vi "Main.vi"() -> ()   [LabVIEW 2017]
uses:
  type defs/action buttons.ctl
  type defs/mode buttons.ctl
  <vilib>/vision/Pattern Matching.llb/IMAQ GM Match Report.ctl
  type defs/states.ctl
  type defs/data.ctl
  <vilib>/vision/Image Controls.llb/IMAQ Image.ctl
  <vilib>/myRIO/Instrument Drivers/Onboard IO/PWM/typedefs/PWM Reference.ctl
  <vilib>/myRIO/Common/Instrument Driver Framework/Utilities/typedefs/myRIO Generic Hardware Reference.ctl
  <vilib>/myRIO/Common/Instrument Driver Framework/Utilities/typedefs/Hardware Version Enum.ctl
  <vilib>/myRIO/Common/Instrument Driver Framework/Utilities/typedefs/myRIO v1.0 Reference.ctl
  <vilib>/myRIO/Common/Instrument Driver Framework/Utilities/typedefs/Generic FPGA Reference.ctl
  <vilib>/myRIO/Common/Instrument Driver Framework/myRIO v1.0/PWM/typedefs/PWM Channels Enum.ctl
  <vilib>/myRIO/Instrument Drivers/Onboard IO/PWM/typedefs/PWM Configuration.ctl
  <vilib>/userdefined/High Color/nirio_resource_hc.ctl
  <vilib>/myRIO/Instrument Drivers/Onboard IO/DIO/typedefs/DIO Reference.ctl
  <vilib>/myRIO/Common/Instrument Driver Framework/myRIO v1.0/DIO/typedefs/DIO Channels List.ctl
  <vilib>/myRIO/Common/Instrument Driver Framework/myRIO v1.0/DIO/typedefs/DIO Channels Enum.ctl
  type defs/task.ctl
  <vilib>/myRIO/Common/Instrument Driver Framework/Utilities/vis/Is FPGA Ref Available.vi
  <vilib>/myRIO/Common/Instrument Driver Framework/myRIO v1.0/PWM/vis/myRIO v1.1 Open PWM.vi
  <vilib>/myRIO/Instrument Drivers/Onboard IO/PWM/vis/Set Duty Cycle and Frequency.vi
  <vilib>/myRIO/Common/Instrument Driver Framework/myRIO v1.0/DIO/vis/myRIO v1.1 Open DIO.vi
  <vilib>/myRIO/Instrument Drivers/Onboard IO/DIO/vis/Write.vi
  <vilib>/myRIO/Instrument Drivers/Onboard IO/DIO/vis/Read.vi
  <vilib>/myRIO/Common/Instrument Driver Framework/Utilities/vis/Validate Channels.vi
  <vilib>/myRIO/Common/Instrument Driver Framework/myRIO v1.0/PWM/vis/myRIO v1.0 Reserve PWM.vi
  <vilib>/myRIO/Common/Instrument Driver Framework/myRIO v1.0/DIO/vis/myRIO v1.0 Reserve DIO.vi
  <vilib>/myRIO/Common/Instrument Driver Framework/myRIO v1.0/UART/vis/myRIO v1.0 Close UART.vi
  <vilib>/myRIO/Common/Instrument Driver Framework/myRIO v1.0/PWM/vis/myRIO v1.0 Build MUX Configuration PWM.vi
  <vilib>/myRIO/Common/Instrument Driver Framework/myRIO v1.0/Resource Manager/vis/myRIO v1.0 Reserve Channel List.vi
  <vilib>/myRIO/Common/Instrument Driver Framework/myRIO v1.0/DIO/vis/myRIO v1.0 Build MUX Configuration DIO.vi
  <vilib>/myRIO/Common/Instrument Driver Framework/myRIO v1.0/Resource Manager/vis/myRIO v1.0 Create Configuration List.vi
  <vilib>/myRIO/Common/Instrument Driver Framework/myRIO v1.0/Resource Manager/vis/myRIO v1.0 Reserve Channel.vi
  <vilib>/myRIO/Common/Instrument Driver Framework/myRIO v1.0/Resource Manager/vis/myRIO v1.0 Unreserve Channel.vi
  <vilib>/myRIO/Common/Instrument Driver Framework/myRIO v1.0/Resource Manager/vis/myRIO v1.0 Build Mutex Name.vi
  <vilib>/Utility/VariantDataType/GetNumericInfo.vi
  <vilib>/Utility/error.llb/Error Cluster From Error Code.vi
  <vilib>/myRIO/Common/Instrument Driver Framework/myRIO v1.0/myRIO v1.1 Open.vi
  <vilib>/myRIO/Common/Instrument Driver Framework/Utilities/vis/IO Manager.vi
  <vilib>/myRIO/Common/Instrument Driver Framework/Utilities/vis/Configuration Manager.vi
  <vilib>/myRIO/Common/Instrument Driver Framework/myRIO v1.0/Resource Manager/vis/myRIO v1.0 Configure IO.vi
  <vilib>/myRIO/Common/Instrument Driver Framework/myRIO v1.0/myRIO v1.0 Close.vi
  <vilib>/myRIO/Common/Instrument Driver Framework/myRIO v1.0/PWM/vis/myRIO v1.0 Write PWM.vi
  <vilib>/myRIO/Common/Instrument Driver Framework/myRIO v1.0/DIO/vis/myRIO v1.0 Write DIO.vi
  <vilib>/myRIO/Common/Instrument Driver Framework/myRIO v1.0/DIO/vis/myRIO v1.0 Read DIO.vi
  <vilib>/myRIO/Common/Instrument Driver Framework/Utilities/vis/FPGA Ref Manager.vi
  <vilib>/myRIO/Common/Instrument Driver Framework/myRIO v1.0/myRIO v1.0 Reset FPGA.vi
  <vilib>/myRIO/Common/Instrument Driver Framework/myRIO v1.0/IRQ/vis/myRIO v1.0 IRQ Info FGV.vi
  <vilib>/myRIO/Common/Instrument Driver Framework/myRIO v1.0/IRQ/vis/myRIO v1.0 Timer IRQ Info FGV.vi
  <vilib>/myRIO/Common/Instrument Driver Framework/myRIO v1.0/IRQ/vis/myRIO v1.0 ISR Agent.vi
  <vilib>/myRIO/Express VI/Onboard IO/PWM/PWM Express VI.xnode
  <vilib>/myRIO/Instrument Drivers/Onboard IO/PWM/vis/myRIO PWM Open.xnode
  <vilib>/myRIO/Express VI/Onboard IO/DO/DO Express VI.xnode
  <vilib>/myRIO/Instrument Drivers/Onboard IO/DIO/vis/myRIO DIO Open.xnode
  <vilib>/myRIO/Express VI/Onboard Devices/LED/LED Express VI.xnode
  <vilib>/myRIO/Express VI/Onboard Devices/Button/Button Express VI.xnode
  <vilib>/vision/NI_Vision_Development_Module.lvlib
  <vilib>/myRIO/Instrument Drivers/Onboard IO/DIO/DIO.lvlib
  <vilib>/myRIO/Instrument Drivers/Onboard IO/PWM/PWM.lvlib
  <vilib>/myRIO/Instrument Drivers/Utilities/Utilities.lvlib
panel:
  in  "ROI Descriptor COLOR":T1={"Global Rectangle"=[86, 71, 180, 164], "Contours"=[{"ID"=enum."External", "Type"=3, "Coordinates"=[86, 71, 180, 164]}]} {"Contours"."Type" items=["No Selection", "Point", "Line", "Rectangle", "Oval", "Polygon", "Freehand Region", "Annulus", "Unused2", "Unused3", "Broken Line", "Freehand Line", "Rotated Rectangle"]}
  out "y0 (circle)":i32
  out "x0 (circle)":i32
  out "x1 (circle)":i32
  out "y1 (circle)":i32
  in  "divider (circle)":dbl=1.0
  out "error out 2":errorcluster
  out "___Test___":i32[](array[numeric])
  in  "Ball index":i32=1
  out "CircleRadius":dbl
  in  "Look at ball":bool
  in  "x = y?":bool
  in  "y":sgl=1.0
  out "Scale":sgl
  out "error out":errorcluster
  in  "Tab Control":enum32{"Motors", "Shape/Color", "Pattern"}(tab)
  in  "Left+":bool
  in  "Left-":bool
  in  "Right+":bool
  in  "Right-":bool
  in  "M+":bool
  in  "M-":bool
  in  "G+":bool
  in  "G-":bool
  in  "M_PWM":dbl=0.5
  in  "L_PWM":dbl=0.5
  in  "R_PWM":dbl=0.5
  in  "M+ (onGrab)":bool
  out "Circles Calibrated (Shape Detection 1)":T2(array[cluster]) {"Position"."Y" format="%.2f"; "Position"."X" format="%.2f"}
  out "Number of Matches (Shape Detection 1)":i32
  out "Color":i32
  in  "Circle Descriptor (Shape Detection 1)":cluster{"Min Radius":dbl, "Max Radius":dbl}={"Min Radius"=16.0, "Max Radius"=500.0}
  in  "Align X - t, Y - f":bool
  in  "grab time (ms)":u32
  out "Class (Particle Classification 1)":string
  out "y0":i32
  out "x0":i32
  out "x1":i32
  out "y1":i32
  out "Number of Matches (Geometric Matching 1)":i32
  out "Calibrated Matches (Geometric Matching 1)":T3[](array[typedef]) {"Correlation Score" format="%.2f"; "Target Template Curve Score" format="%.2f"; "Template Target Curve Score" format="%.2f"; "Bounding Box"."y" format="%.2f"; "Bounding Box"."x" format="%.2f"; "Position"."y" format="%.2f"; "Position"."x" format="%.2f"; "Score" format="%.2f"; "Scale" format="%.2f"; "Angle" format="%.2f"; "Occlusion %" format="%.2f"}
  out "curY":dbl
  out "curX":dbl
  out "Y is in range":bool
  out "X is in range":bool
  in  "defY":dbl=170.0
  in  "Range":dbl=40.0
  in  "defX":dbl=150.0
  in  "mode buttons":T4
  out "image display":T5(plugin-control)
  in  "action buttons":T6
  in  "Stop":bool
  # "Machine\nVision\nApp"
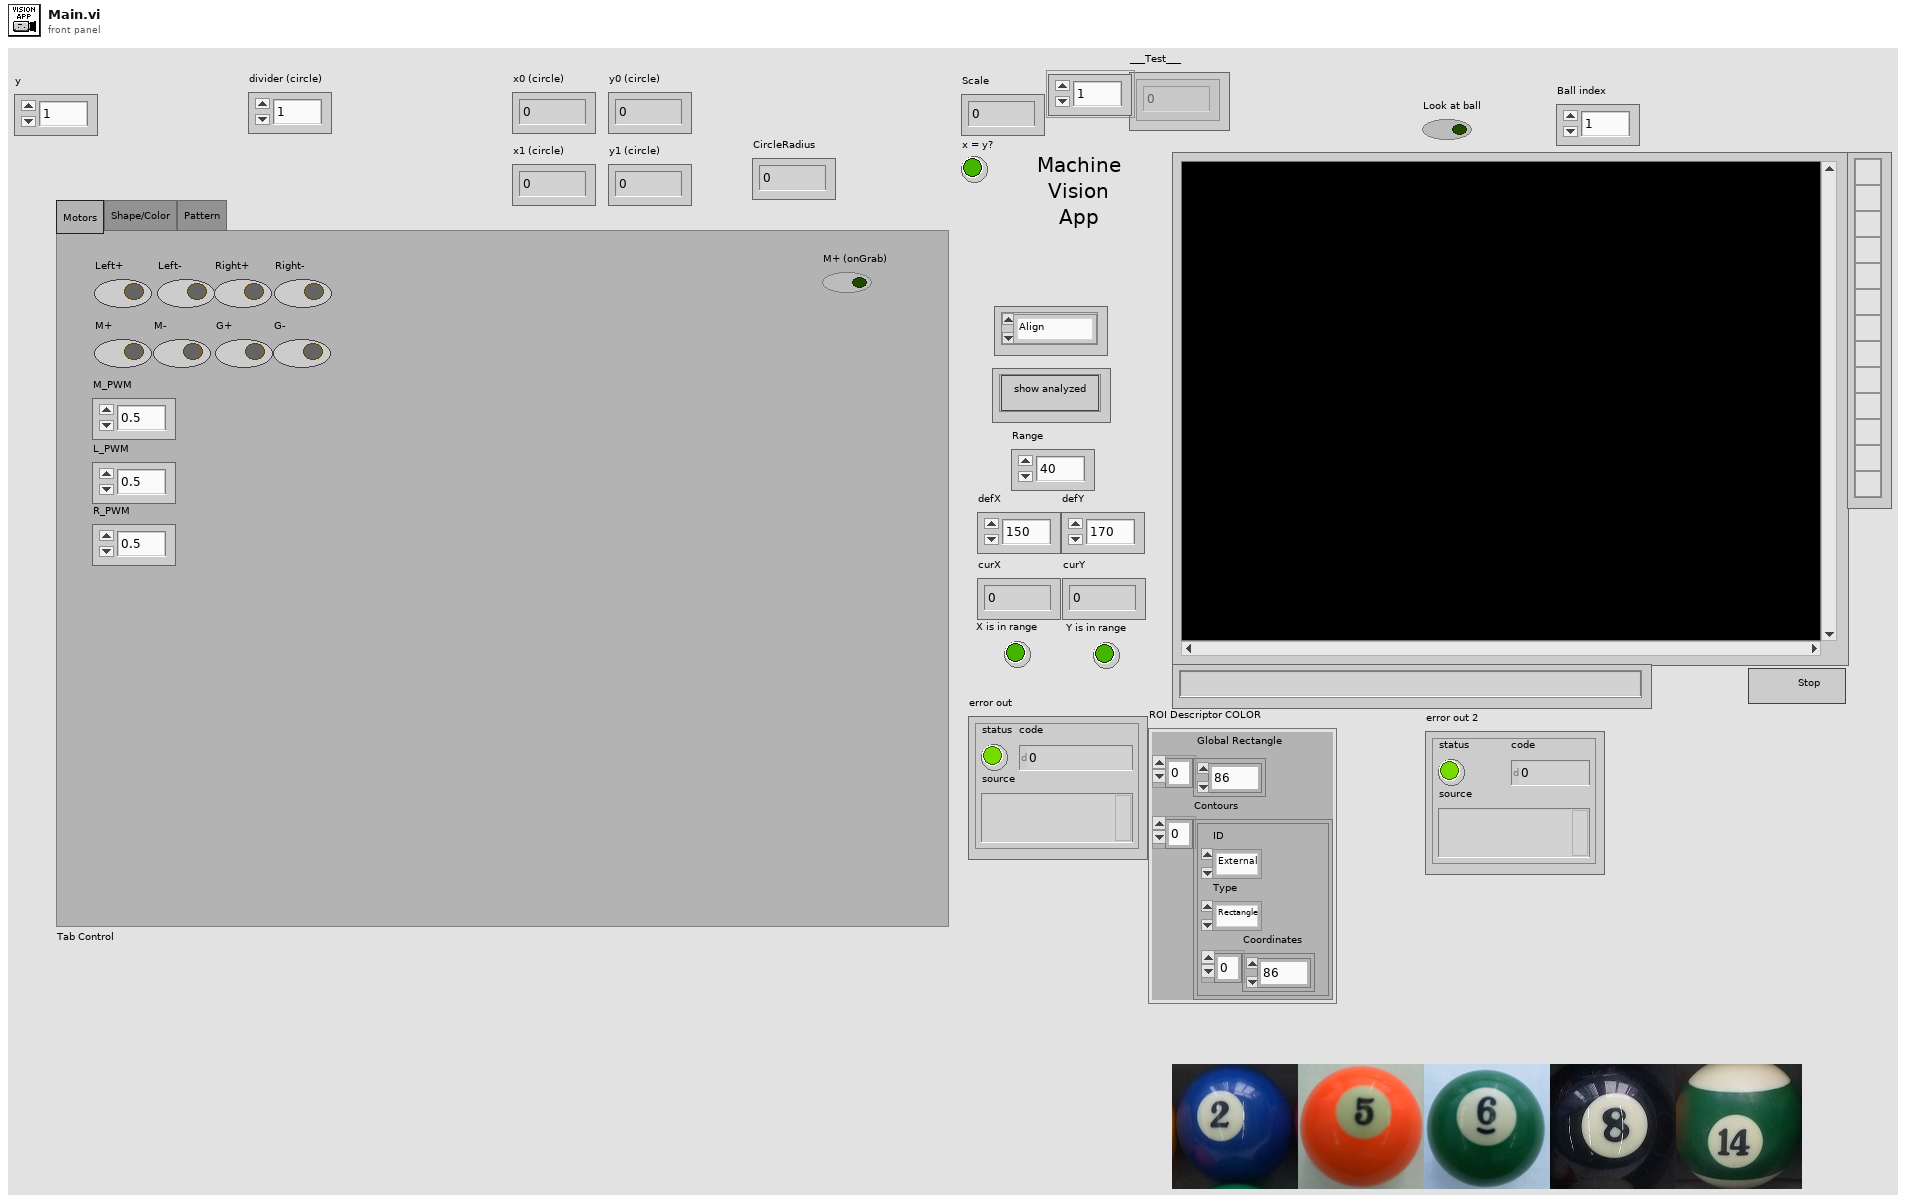
[diagram p1: front panel]
types:
  T1 = cluster{"Global Rectangle":i32[], "Contours":cluster{"ID":enum32{"External", "Internal"}, "Type":u32, "Coordinates":i32[]}[]}
  T2 = cluster{"Position":cluster{"X":sgl, "Y":sgl}, "Radius":dbl, "Score":dbl}[]
  T3 = typedef "IMAQ GM Match Report.ctl" = cluster{"Position":cluster{"x":sgl, "y":sgl}, "Angle":sgl, "Scale":sgl, "Score":sgl, "Bounding Box":cluster{"x":sgl, "y":sgl}[], "Contrast Reversed":bool, "Occlusion %":sgl, "Template Target Curve Score":sgl, "Target Template Curve Score":sgl, "Correlation Score":sgl}
  T4 = typedef "mode buttons.ctl" = cluster{"show analyzed":bool}
  T5 = typedef "IMAQ Image.ctl" = refnum<image>
  T6 = typedef "action buttons.ctl" = cluster{"Shape - t, Color - f":enum16{"Align", "Pattern", "Ball", "Other", "Clear", "Joystick control"}}
  T7 = typedef "data.ctl" = cluster{"Shape - t, Color - f":bool, "qsm":cluster{"Webcam image ref":T5, "Analyzed image ref":T5, "Stop webcam":bool}, " image ref":T5, "number img":i32, "ROI Descriptor (Image Mask 1)":cluster{"Global Rectangle":i32[], "Contours":cluster{"ID":enum32{"External", "Internal"}, "Type":u32, "Coordinates":i32[]}[]}, "Pattern class":i32, "Color class":i32, "ROI Descriptor COLOR Mask":cluster{"Global Rectangle":i32[], "Contours":cluster{"ID":enum32{"External", "Internal"}, "Type":u32, "Coordinates":i32[]}[]}, "___Test___":i32[], "ball Positions":i32[]}
  T8 = typedef "states.ctl" = enum16{"(qsm) schedule", "(qsm) initialize", "(qsm) release", "(qsm) clean up", "(qsm) shutdown", "(myRIO) initialize", "(myRIO) clean up", "(myRIO) update ports", "(image) get", "(image) analyze", "(image) show", "(ball) Shape detection", "(ball) Calc ball indx", "(ball) Calculate ROI", "X align", "Wait", "Grab", "(pattern) Find Square", "(pattern) Calculate ROI", "(pattern) Analyze pattern", "(joystick) Joystick control", "Wait for button"}
  T9 = typedef "DIO.lvlib/DIO Reference.ctl" = cluster{"myRIO Reference":T10, "DIO Channels List":T14}
  T10 = typedef "myRIO Generic Hardware Reference.ctl" = cluster{"myRIO Model":T11, "myRIO Hardware Reference":T12}
  T11 = typedef "Hardware Version Enum.ctl" = enum16{"Unknown", "myRIO-1900", "myRIO-1950", "roboRIO", "NI ELVIS RIO CM"}
  T12 = typedef "myRIO v1.0 Reference.ctl" = cluster{"Generic FPGA Reference":T13, "Allow multiple opens":bool}
  T13 = typedef "Generic FPGA Reference.ctl" = refnum<k20>
  T14 = typedef "DIO Channels List.ctl" = T15[]
  T15 = typedef "DIO Channels Enum.ctl" = enum16{"Not Connected", "C/DIO0", "C/DIO1", "C/DIO2", "C/DIO3", "C/DIO4", "C/DIO5", "C/DIO6", "C/DIO7", "A/DIO0", "A/DIO1", "A/DIO2", "A/DIO3", "A/DIO4", "A/DIO5", "A/DIO6", "A/DIO7", "A/DIO8", "A/DIO9", "A/DIO10", "A/DIO11", "A/DIO12", "A/DIO13", "A/DIO14", "A/DIO15", "B/DIO0", "B/DIO1", "B/DIO2", "B/DIO3", "B/DIO4", "B/DIO5", "B/DIO6", "B/DIO7", "B/DIO8", "B/DIO9", "B/DIO10", "B/DIO11", "B/DIO12", "B/DIO13", "B/DIO14", "B/DIO15", "LED0", "LED1", "LED2", "LED3", "Button0", "DIO/DIO0", "DIO/DIO1", "DIO/DIO2", "DIO/DIO3", "DIO/DIO4", "DIO/DIO5", "DIO/DIO6", "DIO/DIO7", "DIO/DIO8", "DIO/DIO9", "SPI/CS0", "SPI/CS1", "SPI/CS2", "SPI/CS3", "LED RADIO (Green)", "LED RADIO (Red)", "LED COMM (Green)", "LED COMM (Red)", "LED MODE (Green)", "LED MODE (Red)"}
  T16 = typedef "nirio_resource_hc.ctl" = tag
  T17 = typedef "PWM.lvlib/PWM Reference.ctl" = cluster{"myRIO Reference":T10, "PWM Channels Enum":T18, "PWM Configuration":T19}
  T18 = typedef "PWM Channels Enum.ctl" = enum16{"Not Connected", "C/PWM0", "C/PWM1", "A/PWM0", "A/PWM1", "A/PWM2", "B/PWM0", "B/PWM1", "B/PWM2", "PWM/PWM0", "PWM/PWM1", "PWM/PWM2", "PWM/PWM3", "PWM/PWM4", "PWM/PWM5", "PWM/PWM6", "PWM/PWM7", "PWM/PWM8", "PWM/PWM9"}
  T19 = typedef "PWM.lvlib/PWM Configuration.ctl" = cluster{"Frequency":dbl, "Duty Cycle":dbl}
  T20 = enum16{"Align", "Pattern", "Ball", "Other", "Clear", "Joystick control"}
  T21 = typedef "task.ctl" = T8[]
  T22 = typedef "Image Type" = u32
  T23 = cluster{"Position":cluster{"X":sgl, "Y":sgl}, "Radius":dbl, "Score":dbl}
  T24 = cluster{"ID":enum32{"External", "Internal"}, "Type":u32, "Coordinates":i32[]}[]
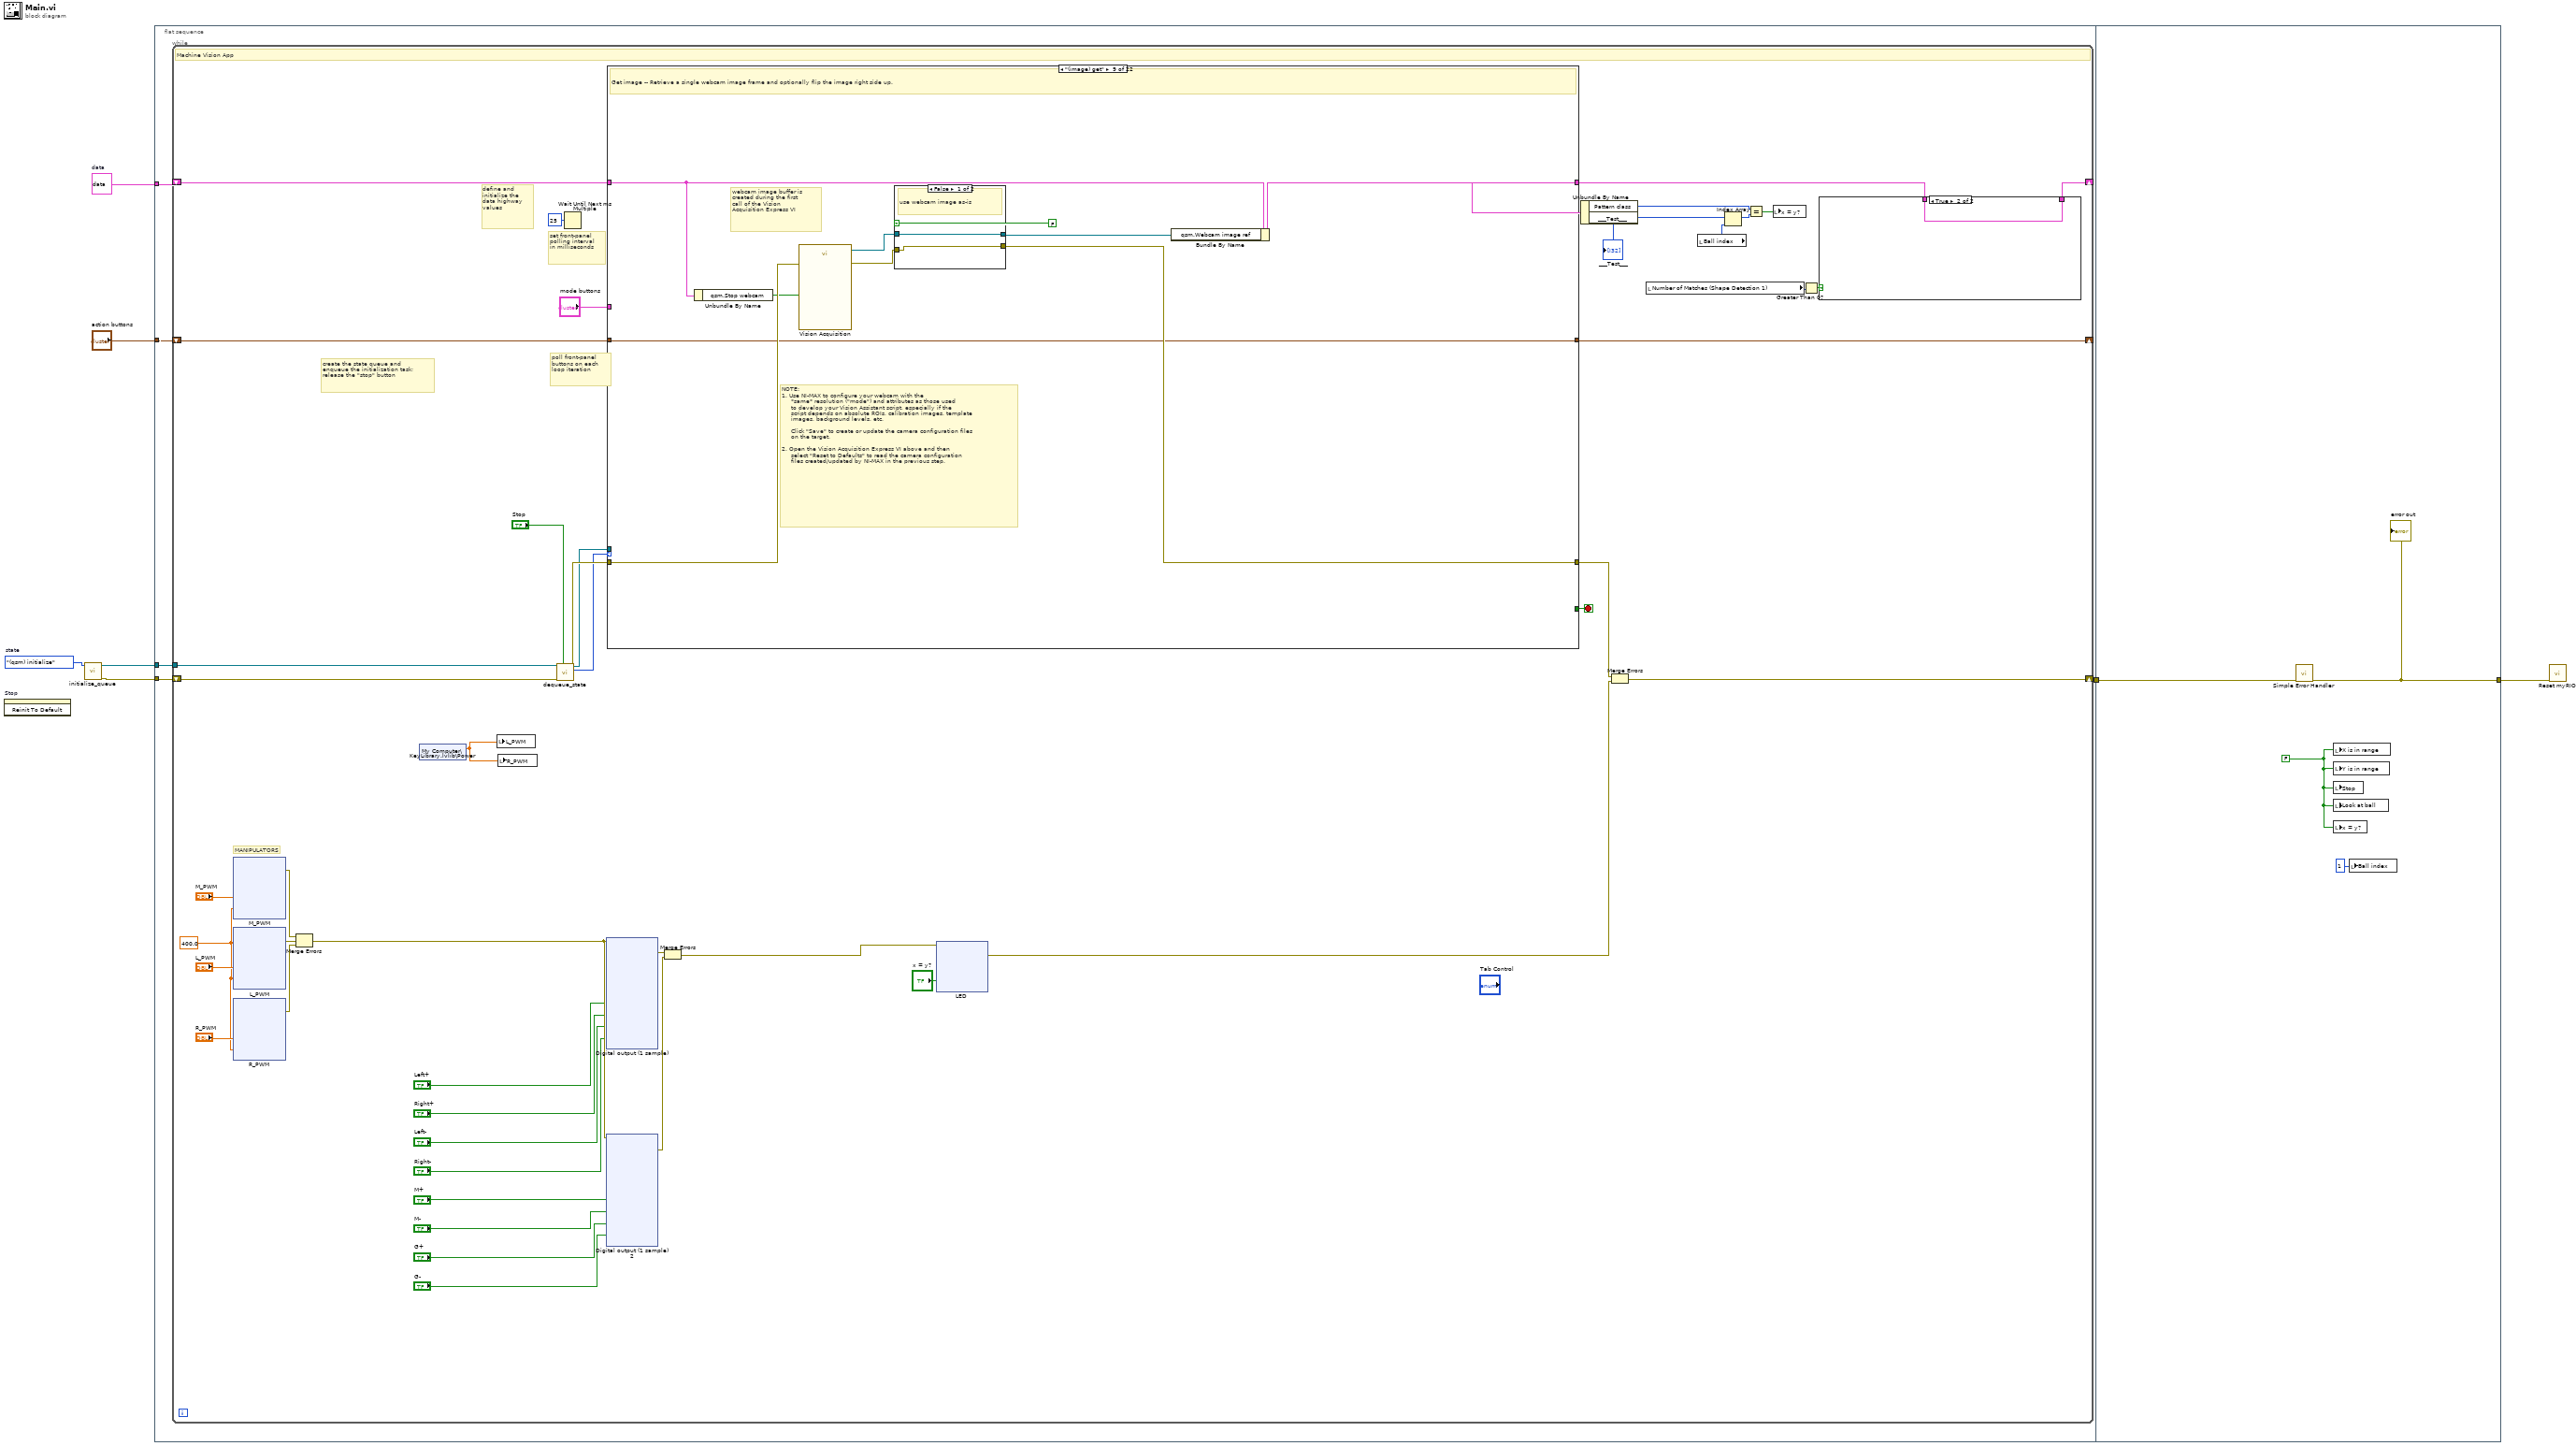
[diagram p0: block diagram]
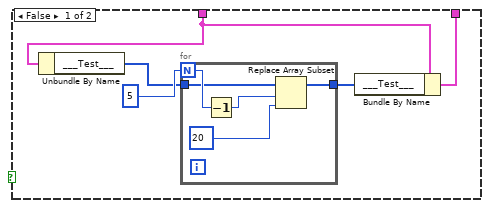
[diagram p2: hidden frame]
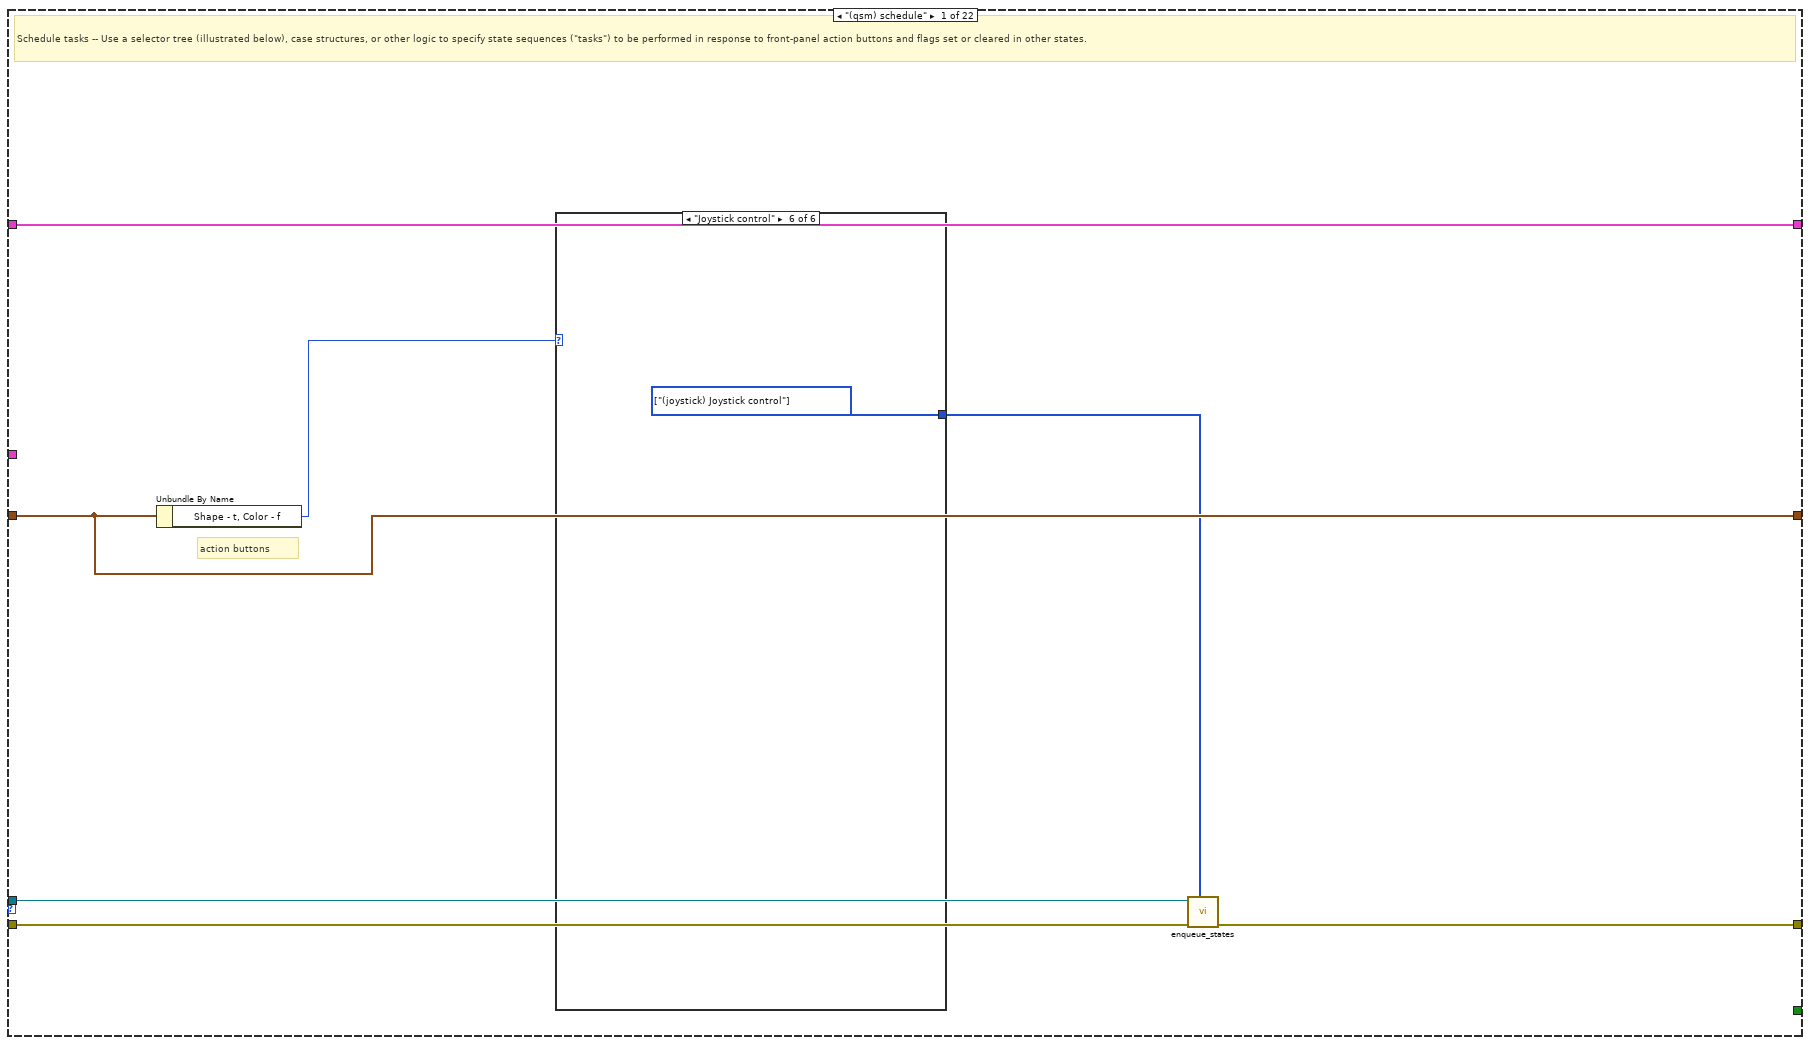
[diagram p3: hidden frame]
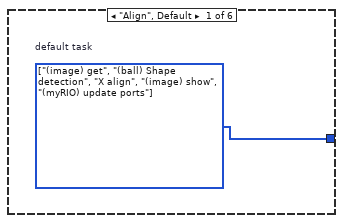
[diagram p4: hidden frame]
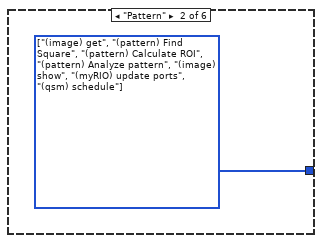
[diagram p5: hidden frame]
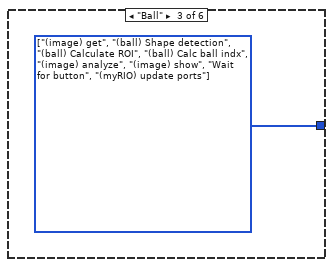
[diagram p6: hidden frame]
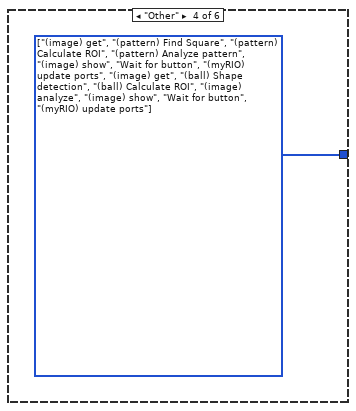
[diagram p7: hidden frame]
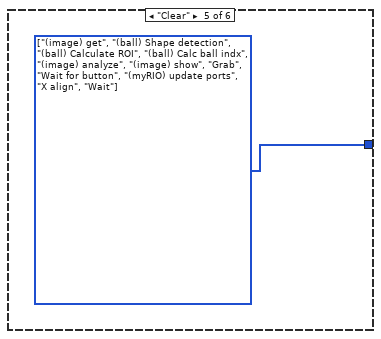
[diagram p8: hidden frame]
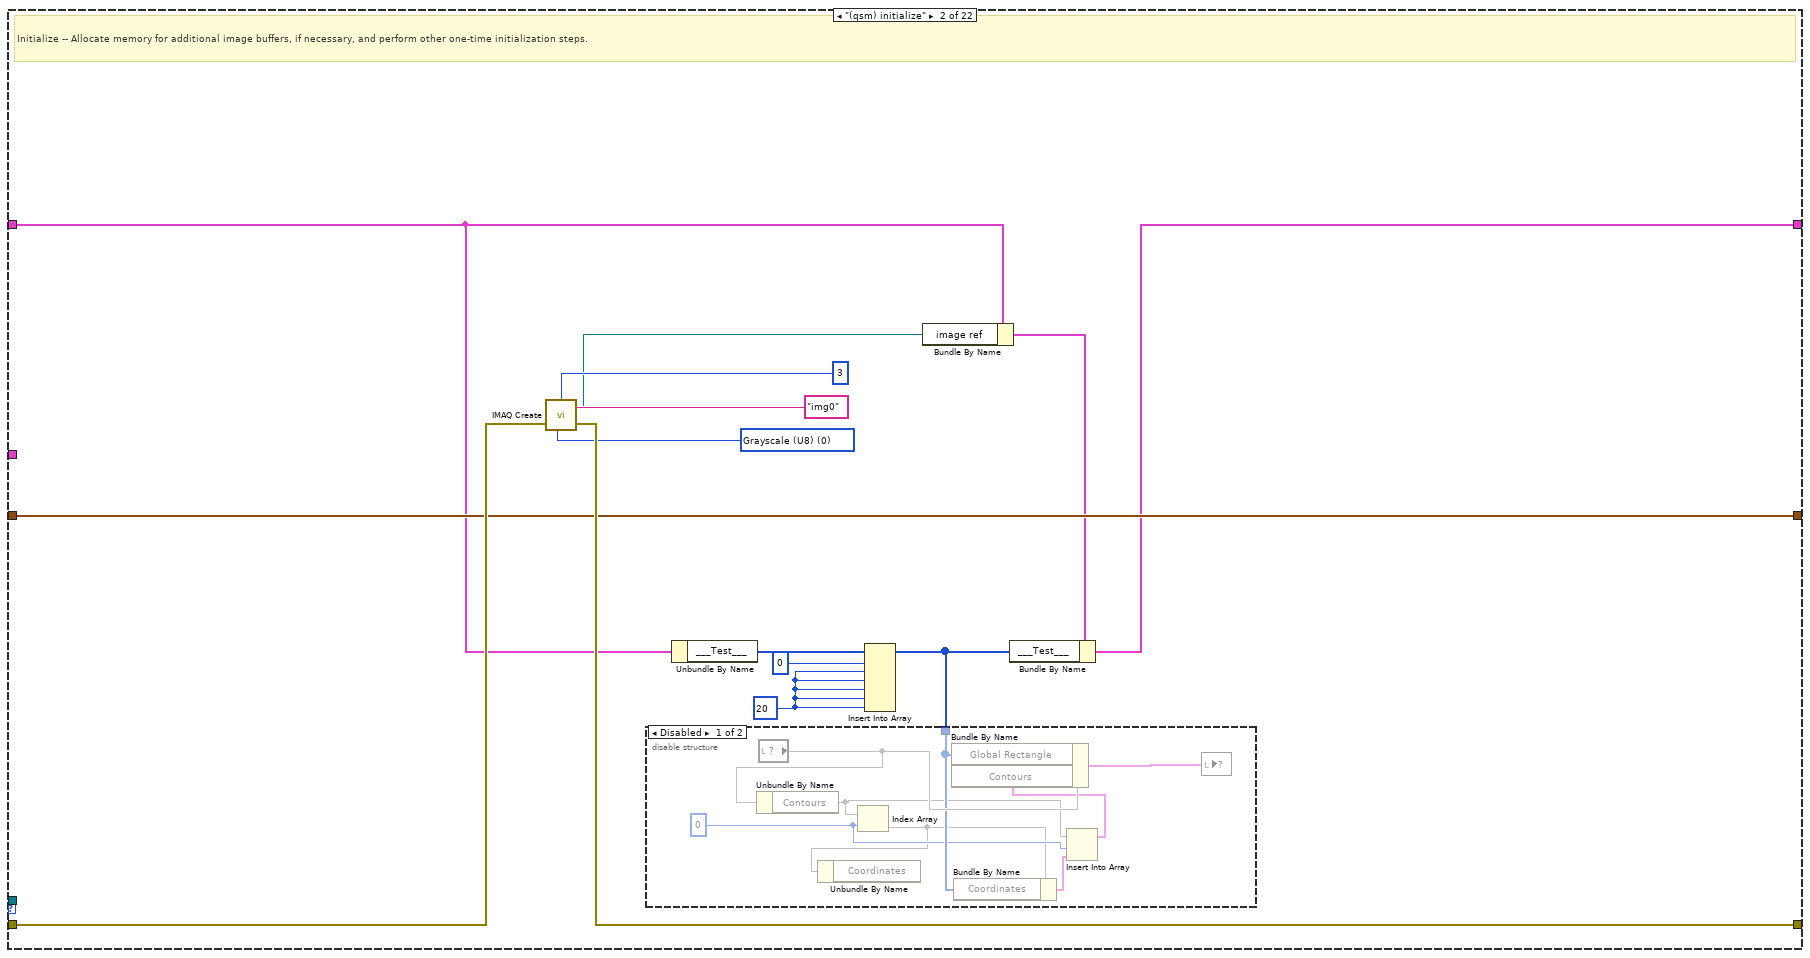
[diagram p9: hidden frame]
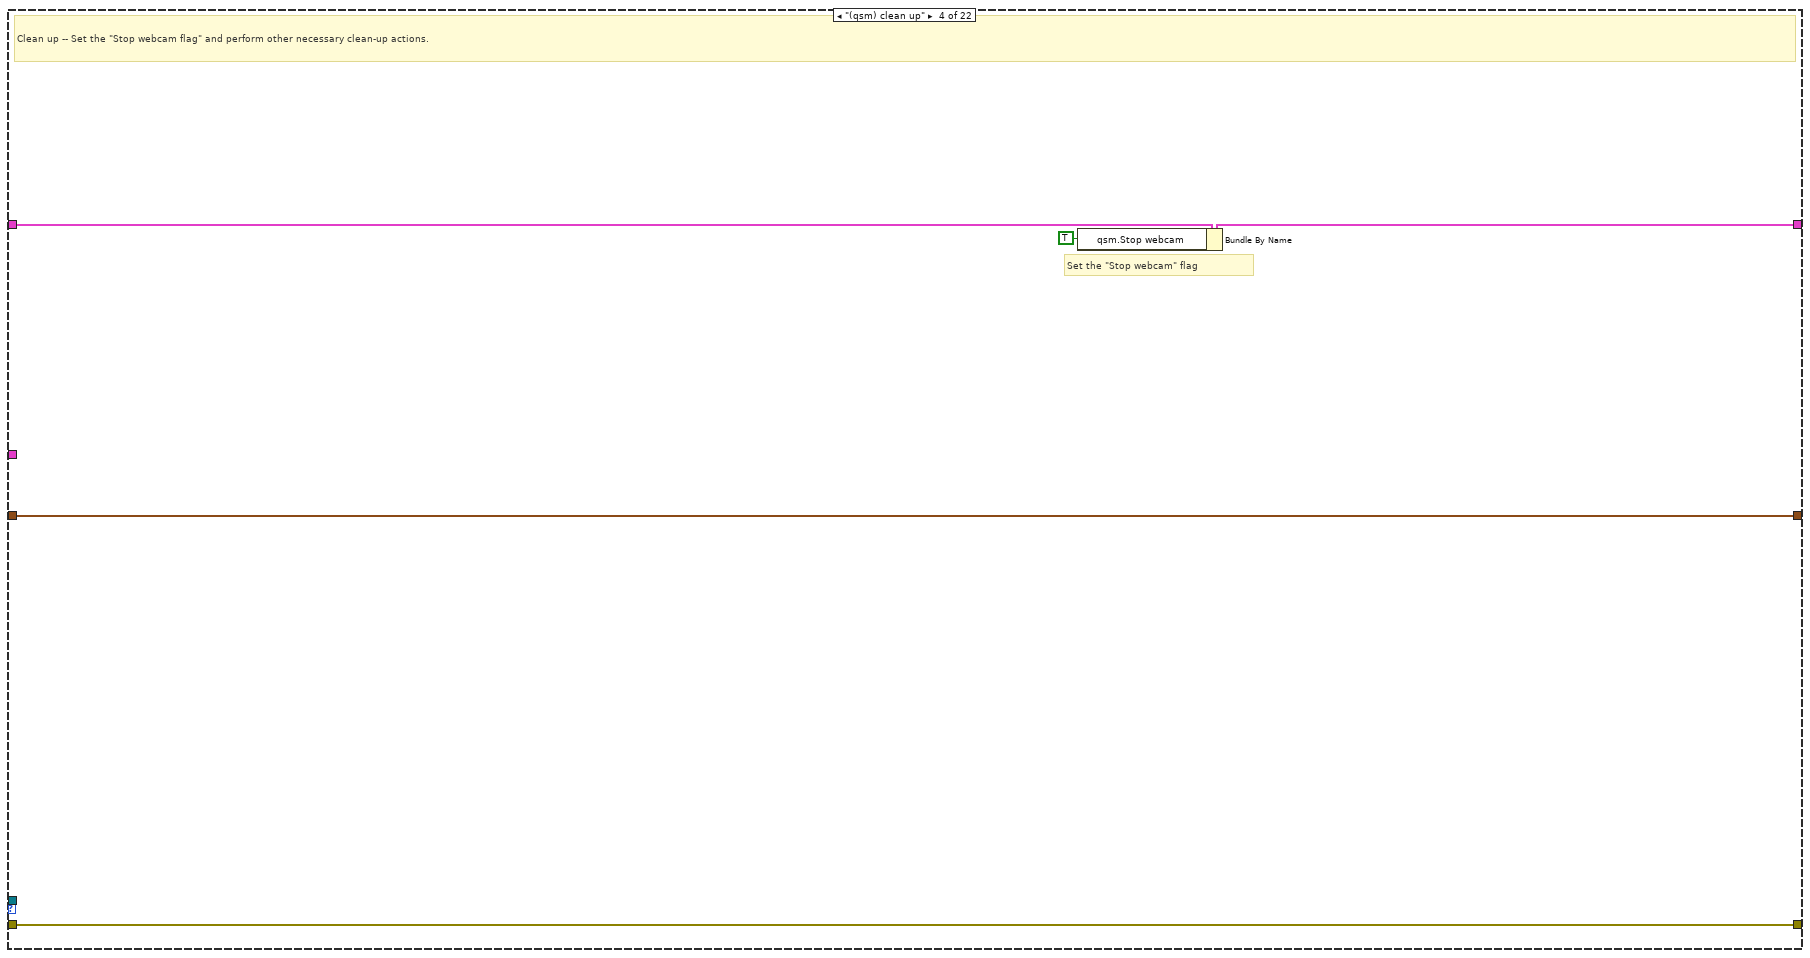
[diagram p12: hidden frame]
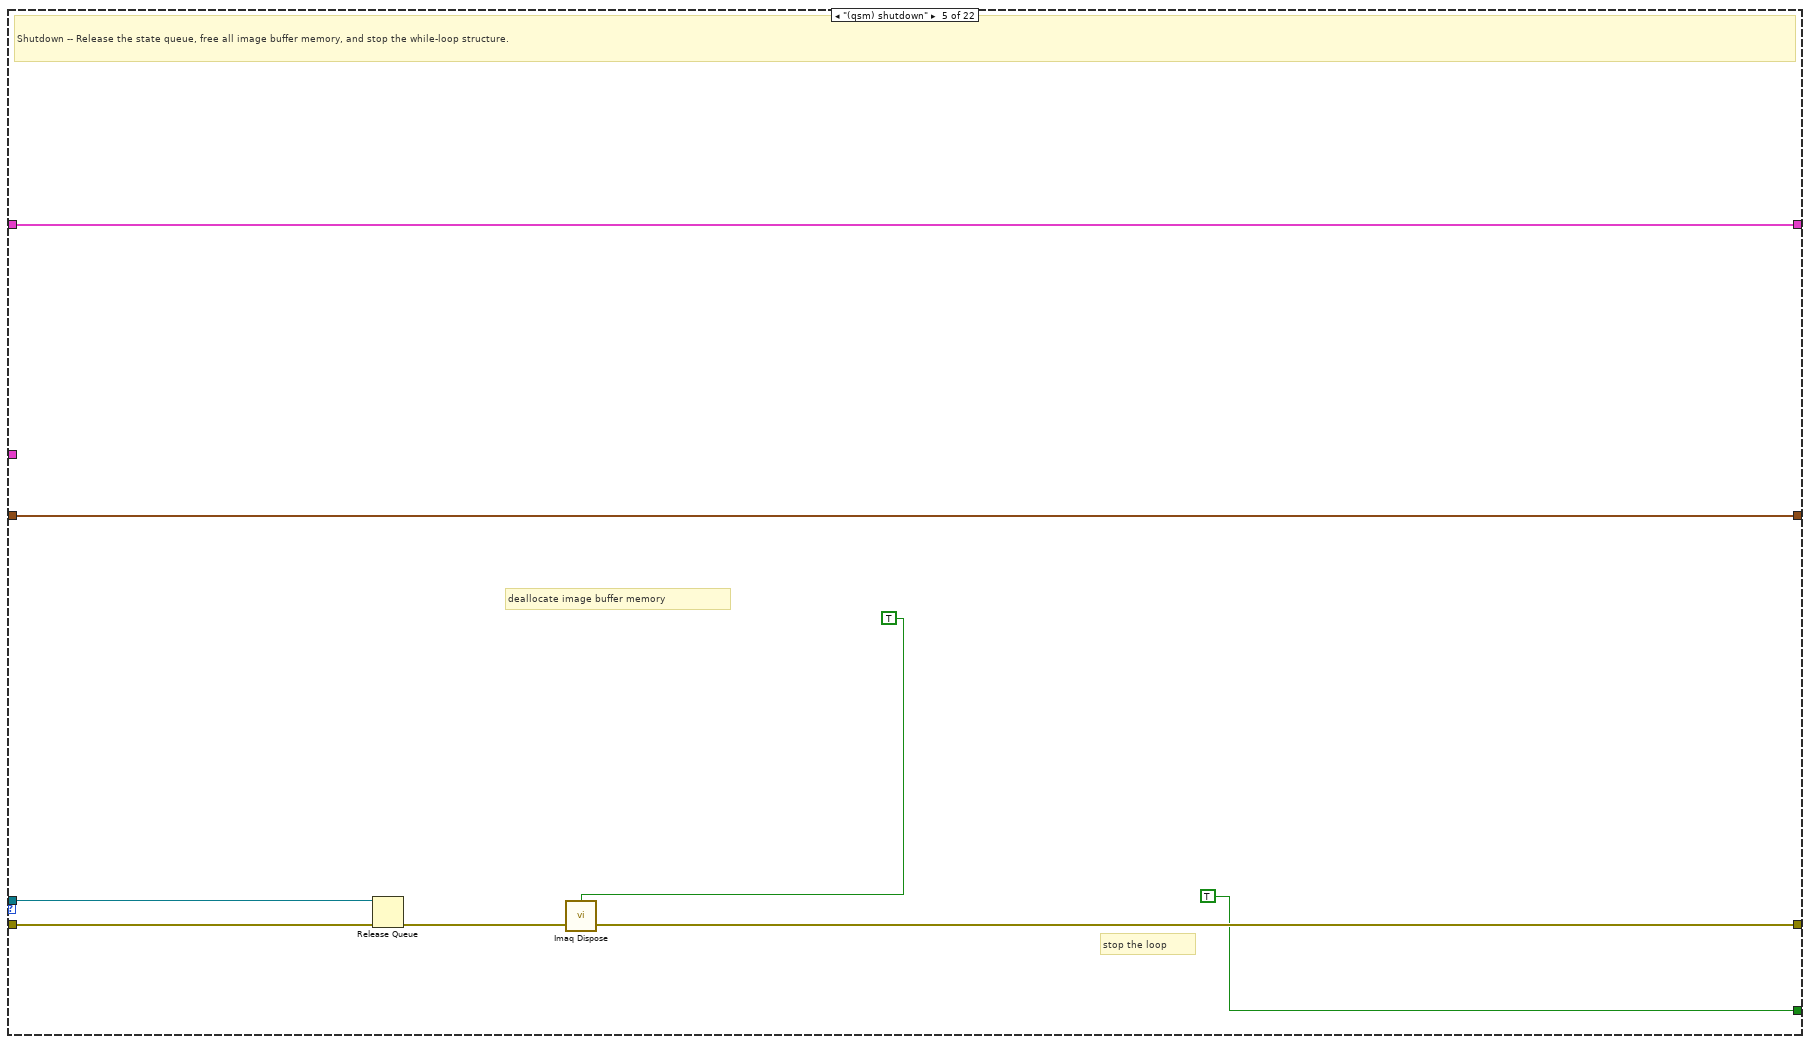
[diagram p13: hidden frame]
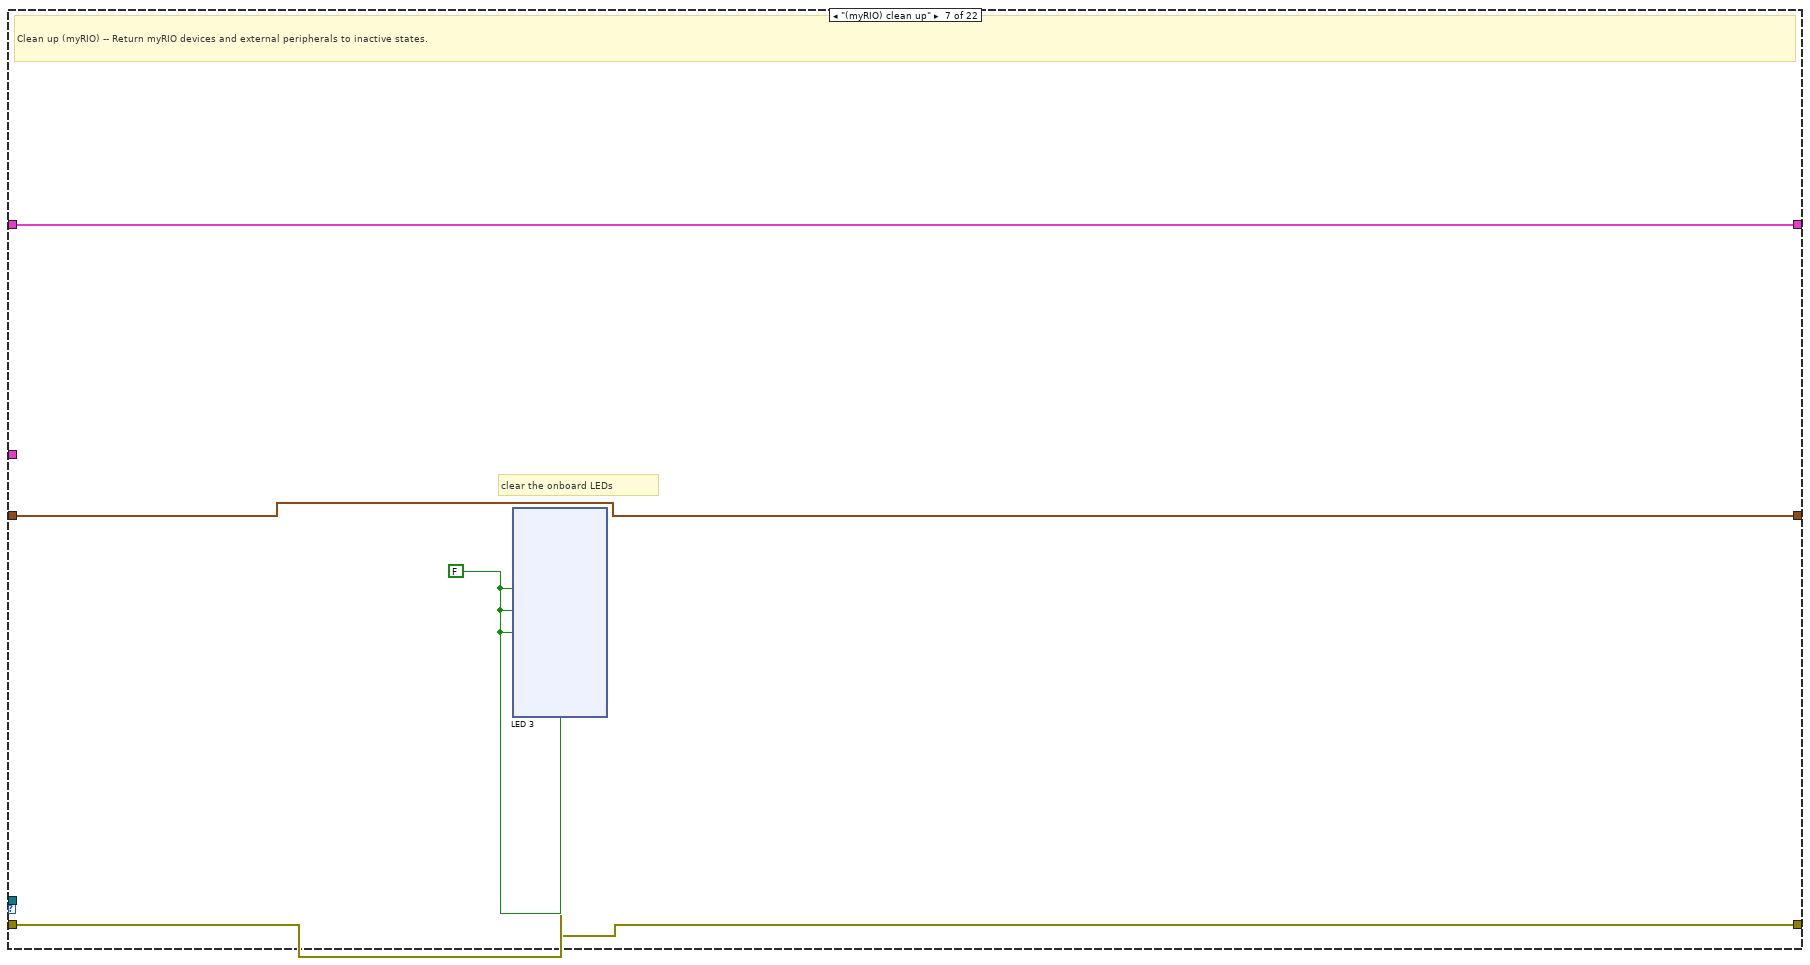
[diagram p15: hidden frame]
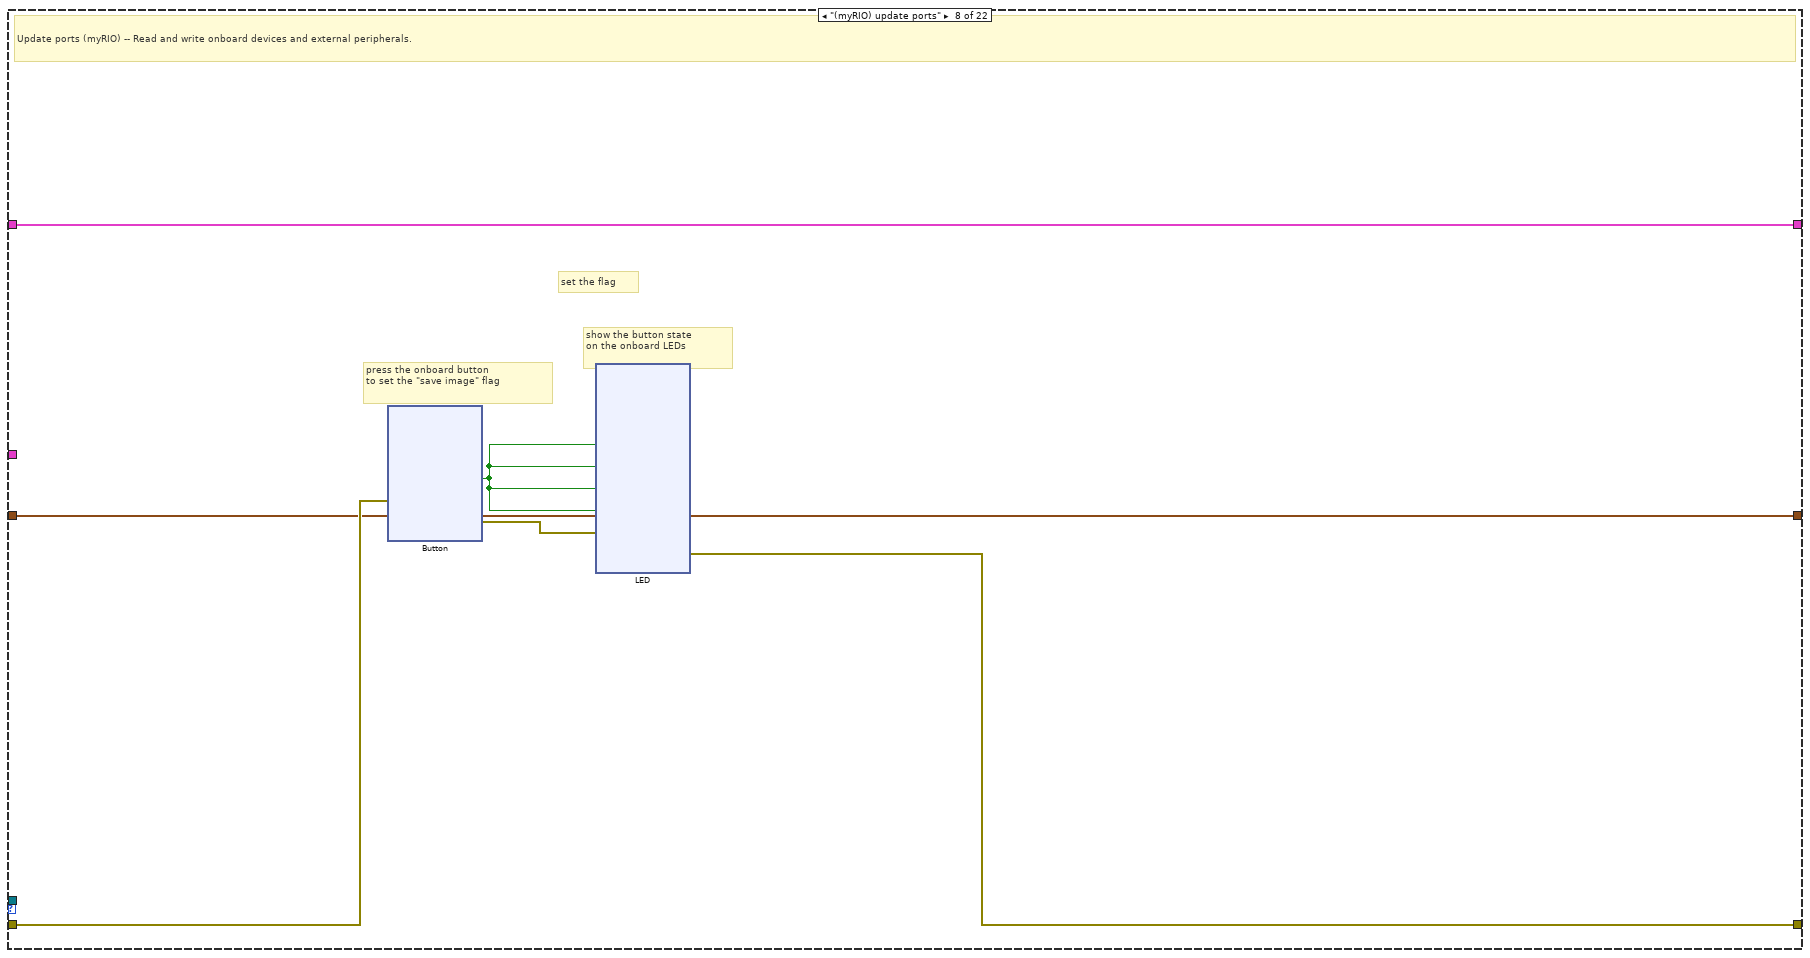
[diagram p16: hidden frame]
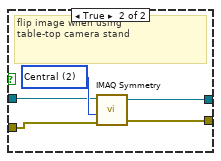
[diagram p17: hidden frame]
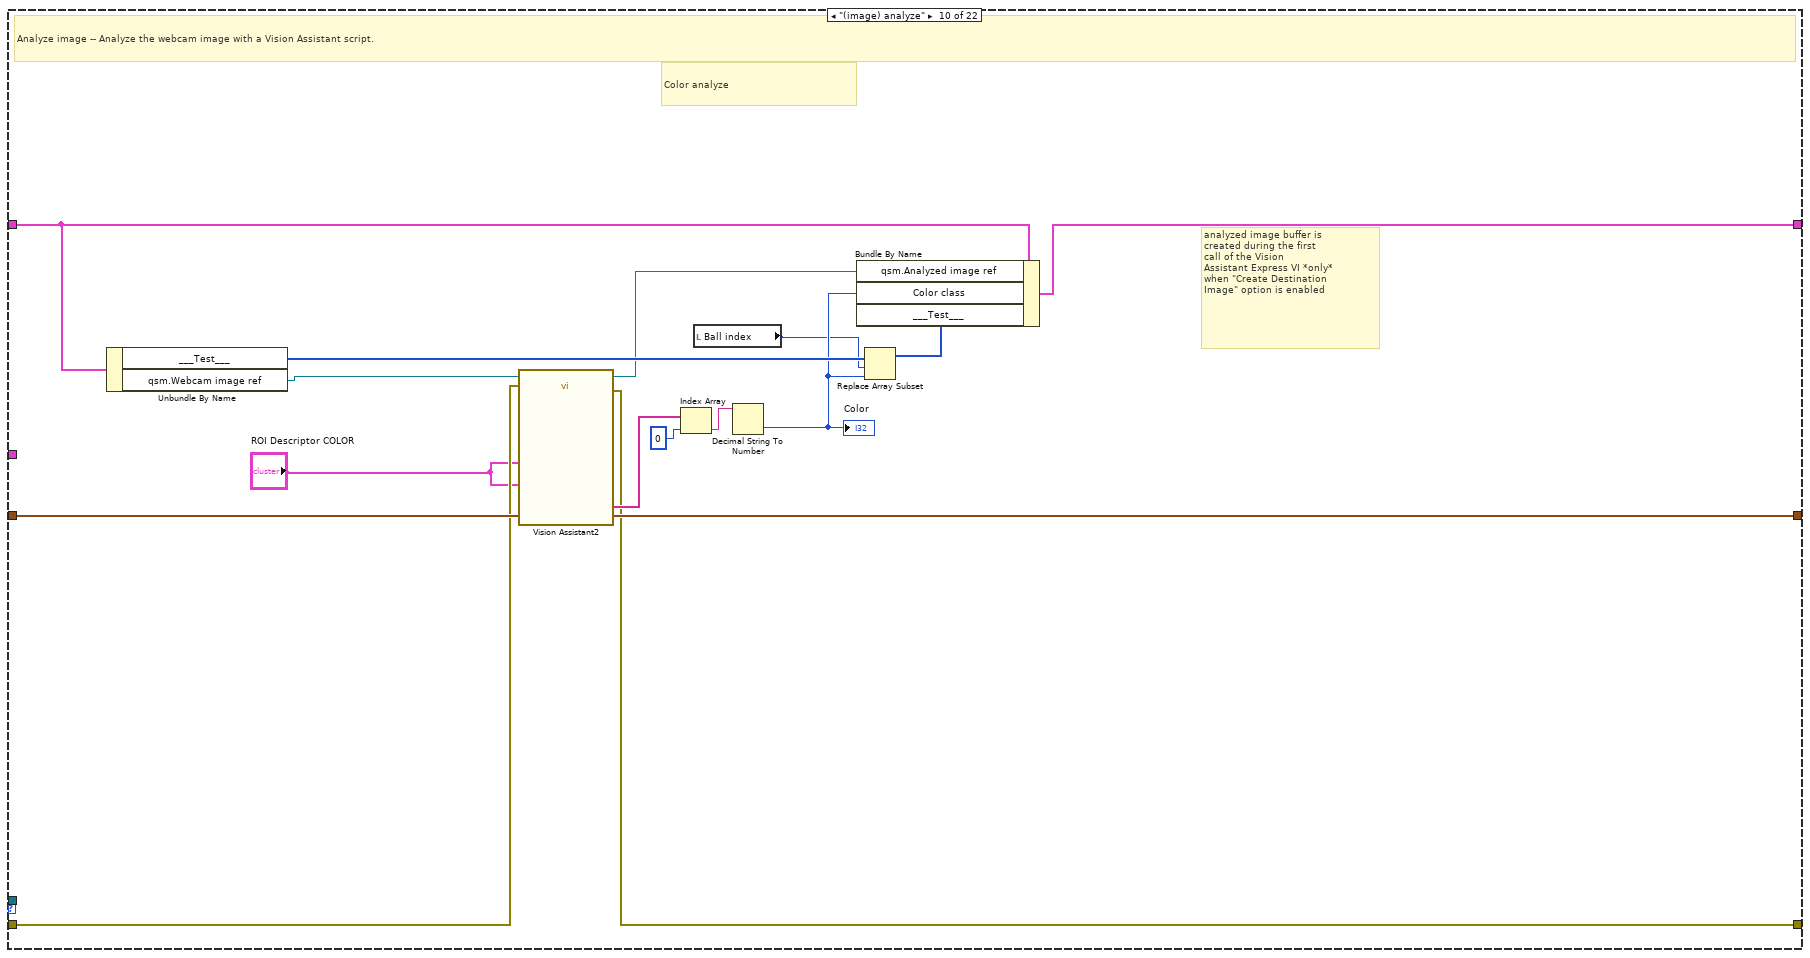
[diagram p18: hidden frame]
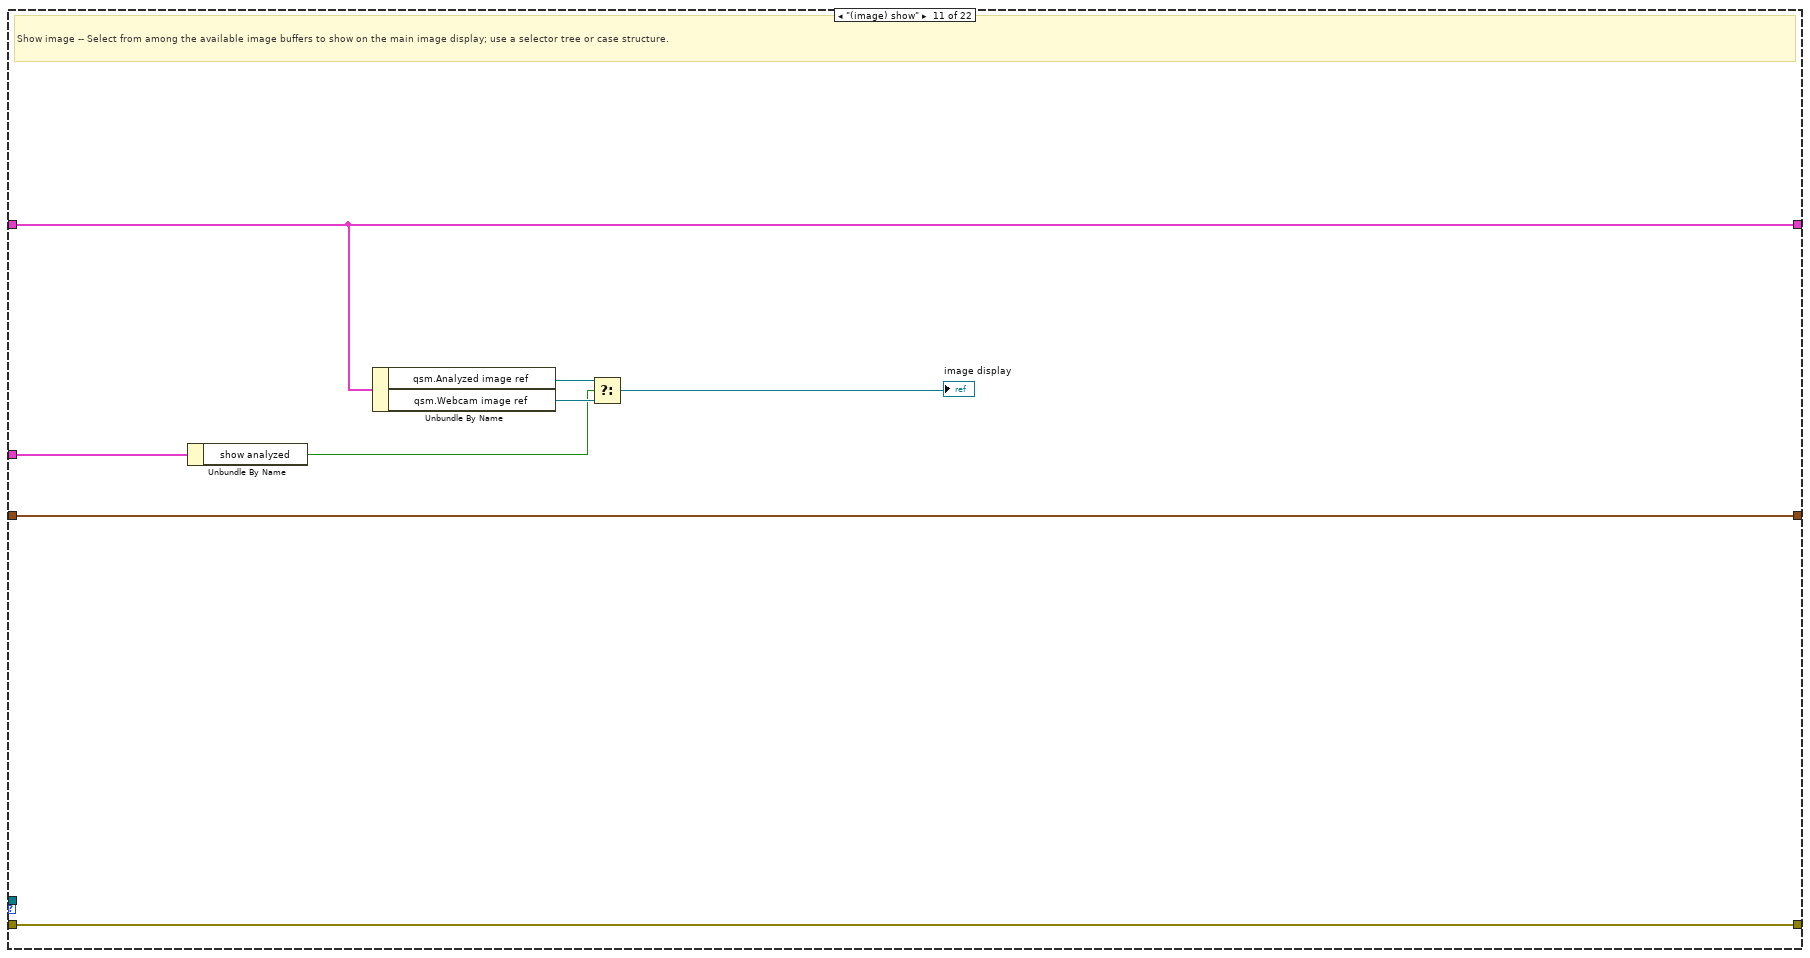
[diagram p19: hidden frame]
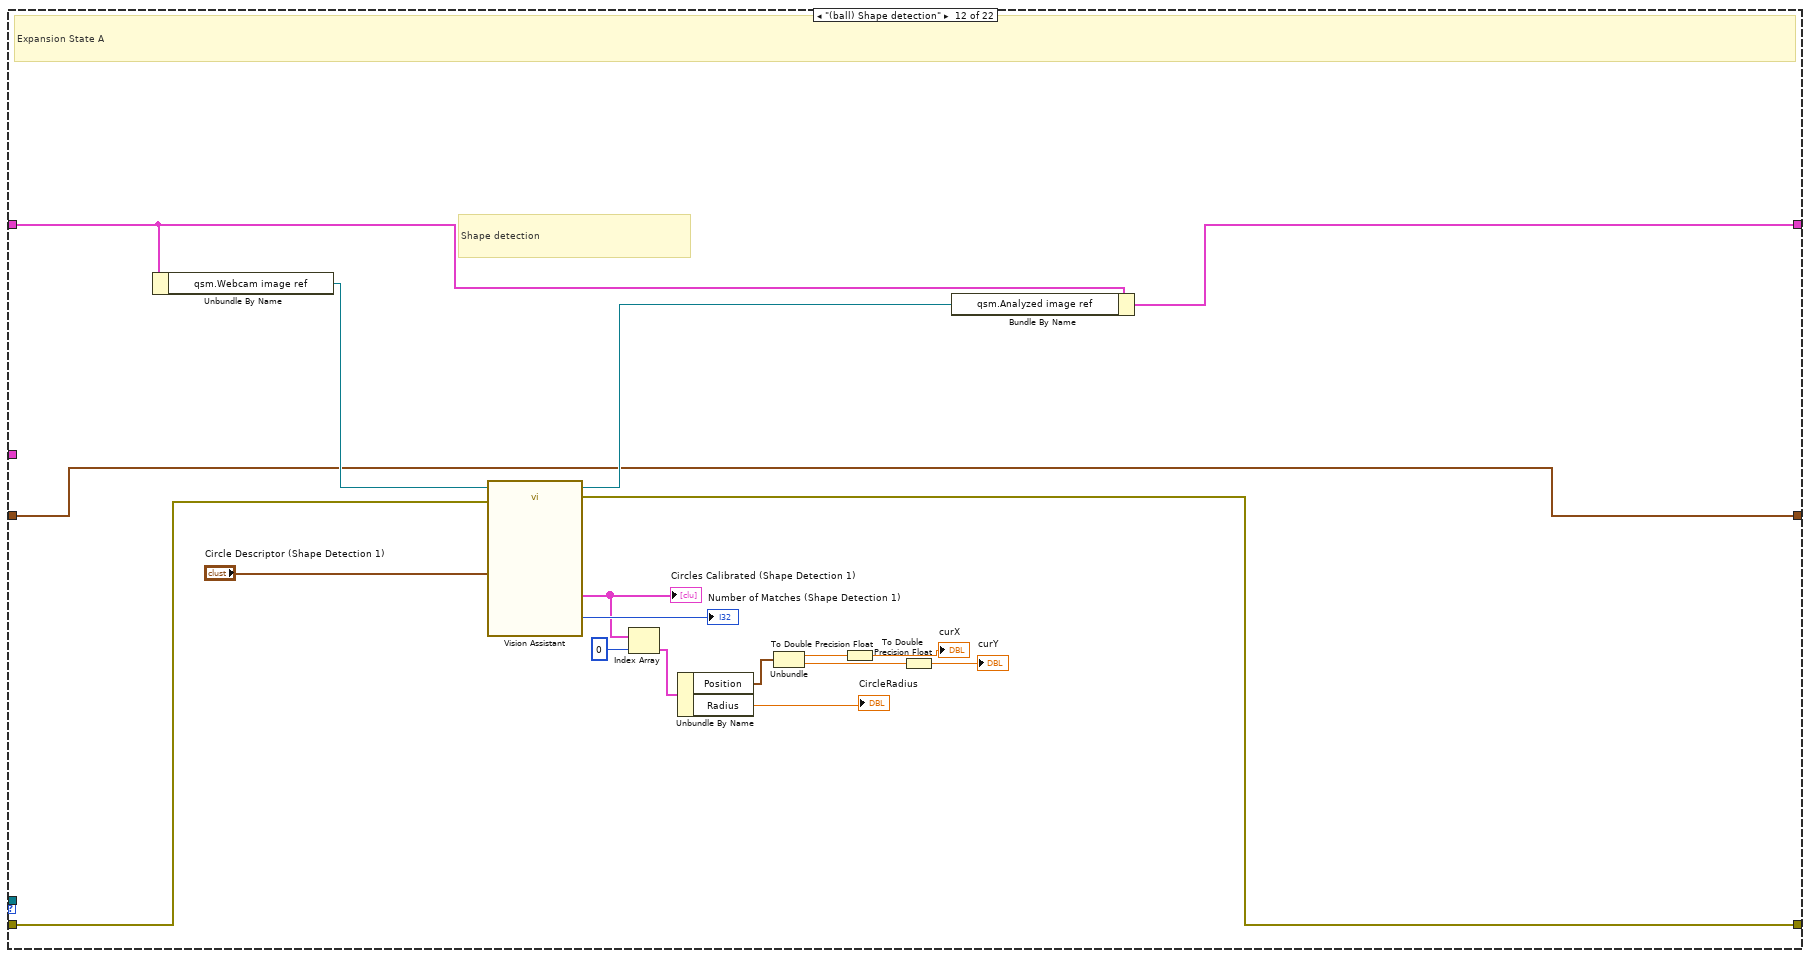
[diagram p20: hidden frame]
diagram:
  w1 = T7 {"Shape - t, Color - f"=FALSE, "qsm"={"Webcam image ref"=refnum, "Analyzed image ref"=refnum, "Stop webcam"=FALSE}, " image ref"=refnum, "number img"=0, "ROI Descriptor (Image Mask 1)"={"Global Rectangle"=[109, 72, 345, 284], "Contours"=[{"ID"=enum."External", "Type"=3, "Coordinates"=[109, 72, 345, 284]}]}, "Pattern class"=0, "Color class"=0, "ROI Descriptor COLOR Mask"={"Global Rectangle"=[51, 157, 345, 350], "Contours"=[{"ID"=enum."External", "Type"=5, "Coordinates"=[137, 230, 93, 226, 75, 199, 49, 200, 56, 145, 98, 111, 200, 119, 250, 126, 235, 166, 240, 212, 188, 243, 303, 244, 336, 247, 336, 271, 335, 292, 335, 318, 314, 323, 293, 334, 279, 345, 272, 349, 187, 349, 186, 335, 120, 334, 112, 314, 100, 297, 59, 291, 51, 288, 51, 287]}]}, "___Test___"=[], "ball Positions"=[]}  # data
  w2 = states."(qsm) initialize"  # state
  n1 = invoke on="Stop" class="Bool (strict)" method="Reinit To Default"() -> ()  [unwired: 3 in, 3 out]
  n2 = call "initialize_queue.vi"("state"=w2) -> ("error out"=w3:errorcluster, "queue out"=w4:refnum<queue>)  [unwired: 9 in]
  n3 = flat-sequence {
    tunnel: [w12] -> w6
    tunnel: "action buttons" -> [w11]
    tunnel: w3 -> [w9]
    tunnel: w4 -> [w10]
    tunnel: w1 -> [w8]
    tunnel: [w644] -> w7
    tunnel: w6 -> [w645]
    frame #0 {
      n4 = while {
        shift-right: [w51] -> w12
        shift-left: w9 -> [w56]
        shift-right: [w21] -> _
        shift-left: w8 -> [w13]
        shift-right: [w32] -> _
        shift-left: w11 -> [w31]
        tunnel: w10 -> [w30]
        stop <- w29 stop-if-true
        w34 = 400.0 ("Frequency [Hz]")
        # "define and \ninitialize the \ndata highway\nvalues"
        # "MANIPULATORS"
        # "create the state queue and\nenqueue the initialization task;\nrelease the \"stop\" button"
        # "set front-panel\npolling interval\nin milliseconds"
        # "poll front-panel\nbuttons on each\nloop iteration"
        # "Machine Vision App"
        n5 = xnode "M_PWM"("Duty Cycle"="M_PWM", "Frequency [Hz]"=w34) -> ("error out"=w50:errorcluster)  [unwired: 1 in]
        n6 = xnode "L_PWM"("Duty Cycle"="L_PWM", "Frequency [Hz]"=w34) -> ("error out"=w49:errorcluster)  [unwired: 1 in]
        n7 = xnode "R_PWM"("Duty Cycle"="R_PWM", "Frequency [Hz]"=w34) -> ("error out"=w48:errorcluster)  [unwired: 1 in]
        n8 = Merge Errors(w50, w49, w48) -> (w45:errorcluster)
        n9 = shared-variable "My Computer\\KeyLibrary.lvlib\\Power"() -> (w14:dbl)  [unwired: 1 in, 1 out]
        n10 = local write "L_PWM"(w14) -> ()
        n11 = local write "R_PWM"(w14) -> ()
        n12 = call "dequeue_state.vi"("stop"="Stop", "error in (no error)"=w56, "queue in"=w30) -> ("error out"=w57:errorcluster, "state"=w52:T8, "queue out"=w33:refnum<queue>)  [unwired: 6 in]
        n13 = Wait Until Next ms Multiple(millisecond multiple=u32 25) -> ()  [unwired: 1 out]
        n14 = xnode "Digital output (1 sample)"("Left+ (A/DIO5 (Pin 21))"="Left+", "Right+ (A/DIO7 (Pin 25))"="Right+", "Left- (A/DIO6 (Pin 23))"="Left-", "Right- (A/DIO13 (Pin 26))"="Right-", "error in (no error)"=w45) -> ("error out"=w47:errorcluster)
        n15 = xnode "Digital output (1 sample) 2"("M+ (B/DIO5 (Pin 21))"="M+", "M- (B/DIO6 (Pin 23))"="M-", "G+ (B/DIO7 (Pin 25))"="G+", "G- (B/DIO13 (Pin 26))"="G-", "error in (no error)"=w45) -> ("error out"=w46:errorcluster)
        n16 = case shown="\"(image) get\"" w52 {
          tunnel: w57 -> [w288 w311 w321 w324 w335 w337 w341 w386 w465 w480 w496 w518 w528 w544 w546 w566 w588 w594 w613 w622 w629 w638]
          tunnel: w33 -> [w289 _ _ _ w334 _ _ _ _ _ _ _ _ _ _ w564 _ _ _ _ _ _]
          tunnel: [w290 w310 w321 w324 w330 w337 w340 w384 w468 w479 w496 w513 w528 w544 w546 w565 w587 w595 w613 w621 w629 w638] -> w18
          tunnel: w31 -> [w287 w305 w320 w323 w329 w336 w339 w382 w461 w489 w493 w509 w527 w542 w545 w568 w589 w599 w611 w617 w634 w639]
          tunnel: w13 -> [w291 w302 w322 w326 w333 w338 w343 w387 w466 w492 w497 w515 w529 w543 w547 w570 w590 w593 w612 w620 w635 w636]
          tunnel: [w291 w303 w322 w325 w333 w338 w343 w387 w470 w491 w497 w514 w529 w543 w547 w569 w590 w592 w600 w619 w635 w636] -> w22
          tunnel: "mode buttons" -> [_ _ _ _ _ _ _ _ _ _ w495 _ _ _ _ _ _ _ _ _ _ _]
          tunnel: [w287 w305 w320 w323 w329 w336 w339 w382 w461 w489 w493 w509 w527 w542 w545 w567 w589 w599 w611 w617 w634 w639] -> w32
          tunnel: [_ _ _ _ TRUE _ _ _ _ _ _ _ _ _ _ _ _ _ _ _ _ _] -> w29
          frame "(qsm) schedule" {
            # "action buttons"
            # "Schedule tasks -- Use a selector tree (illustrated below), case structures, or other logic to specify state sequences (\"tasks\") to be performed in response to front-panel action buttons and flags set or cleared in other states."
            n17 = Unbundle By Name(w287) -> ("Shape - t, Color - f"=w286:T20)
            n18 = case shown="\"Joystick control\"" w286 {
              tunnel: [w292 w293 w294 w295 w296 w297] -> w285
              frame "Align", Default {
                w292 = T21 [enum."(image) get", enum."(ball) Shape detection", enum."X align", enum."(image) show", enum."(myRIO) update ports"] items=["(qsm) schedule", "(qsm) initialize", "(qsm) release", "(qsm) clean up", "(qsm) shutdown", "(myRIO) initialize", "(myRIO) clean up", "(myRIO) update ports", "(image) get", "(image) analyze", "(image) show", "(ball) Shape detection", "(ball) Calc ball indx", "(ball) Calculate ROI", "X align", "Wait", "Grab", "(pattern) Find Square", "(pattern) Calculate ROI", "(pattern) Analyze pattern", "(joystick) Joystick control", "Wait for button"]  # default task
              }
              frame "Pattern" {
                w293 = T21 [enum."(image) get", enum."(pattern) Find Square", enum."(pattern) Calculate ROI", enum."(pattern) Analyze pattern", enum."(image) show", enum."(myRIO) update ports", enum."(qsm) schedule"] items=["(qsm) schedule", "(qsm) initialize", "(qsm) release", "(qsm) clean up", "(qsm) shutdown", "(myRIO) initialize", "(myRIO) clean up", "(myRIO) update ports", "(image) get", "(image) analyze", "(image) show", "(ball) Shape detection", "(ball) Calc ball indx", "(ball) Calculate ROI", "X align", "Wait", "Grab", "(pattern) Find Square", "(pattern) Calculate ROI", "(pattern) Analyze pattern", "(joystick) Joystick control", "Wait for button"] ("task")
              }
              frame "Ball" {
                w294 = T21 [enum."(image) get", enum."(ball) Shape detection", enum."(ball) Calculate ROI", enum."(ball) Calc ball indx", enum."(image) analyze", enum."(image) show", enum."Wait for button", enum."(myRIO) update ports"] items=["(qsm) schedule", "(qsm) initialize", "(qsm) release", "(qsm) clean up", "(qsm) shutdown", "(myRIO) initialize", "(myRIO) clean up", "(myRIO) update ports", "(image) get", "(image) analyze", "(image) show", "(ball) Shape detection", "(ball) Calc ball indx", "(ball) Calculate ROI", "X align", "Wait", "Grab", "(pattern) Find Square", "(pattern) Calculate ROI", "(pattern) Analyze pattern", "(joystick) Joystick control", "Wait for button"] ("task")
              }
              frame "Other" {
                w295 = T21 [enum."(image) get", enum."(pattern) Find Square", enum."(pattern) Calculate ROI", enum."(pattern) Analyze pattern", enum."(image) show", enum."Wait for button", enum."(myRIO) update ports", enum."(image) get", enum."(ball) Shape detection", enum."(ball) Calculate ROI", enum."(image) analyze", enum."(image) show", enum."Wait for button", enum."(myRIO) update ports"] items=["(qsm) schedule", "(qsm) initialize", "(qsm) release", "(qsm) clean up", "(qsm) shutdown", "(myRIO) initialize", "(myRIO) clean up", "(myRIO) update ports", "(image) get", "(image) analyze", "(image) show", "(ball) Shape detection", "(ball) Calc ball indx", "(ball) Calculate ROI", "X align", "Wait", "Grab", "(pattern) Find Square", "(pattern) Calculate ROI", "(pattern) Analyze pattern", "(joystick) Joystick control", "Wait for button"] ("task")
              }
              frame "Clear" {
                w296 = T21 [enum."(image) get", enum."(ball) Shape detection", enum."(ball) Calculate ROI", enum."(ball) Calc ball indx", enum."(image) analyze", enum."(image) show", enum."Grab", enum."Wait for button", enum."(myRIO) update ports", enum."X align", enum."Wait"] items=["(qsm) schedule", "(qsm) initialize", "(qsm) release", "(qsm) clean up", "(qsm) shutdown", "(myRIO) initialize", "(myRIO) clean up", "(myRIO) update ports", "(image) get", "(image) analyze", "(image) show", "(ball) Shape detection", "(ball) Calc ball indx", "(ball) Calculate ROI", "X align", "Wait", "Grab", "(pattern) Find Square", "(pattern) Calculate ROI", "(pattern) Analyze pattern", "(joystick) Joystick control", "Wait for button"] ("task")
              }
              frame "Joystick control" {
                w297 = T21 [enum."(joystick) Joystick control"] items=["(qsm) schedule", "(qsm) initialize", "(qsm) release", "(qsm) clean up", "(qsm) shutdown", "(myRIO) initialize", "(myRIO) clean up", "(myRIO) update ports", "(image) get", "(image) analyze", "(image) show", "(ball) Shape detection", "(ball) Calc ball indx", "(ball) Calculate ROI", "X align", "Wait", "Grab", "(pattern) Find Square", "(pattern) Calculate ROI", "(pattern) Analyze pattern", "(joystick) Joystick control", "Wait for button"]
              }
            }
            n19 = call "enqueue_states.vi"("task"=w285, "error in"=w288, "queue in"=w289) -> ("error out"=w290:errorcluster)  [unwired: 6 in, 1 out]
          }
          frame "(qsm) initialize" {
            w299 = 20
            w308 = T22 0 items=["Grayscale (U8)", "Grayscale (I16)", "Grayscale (SGL)", "Complex (CSG)", "RGB (U32)", "HSL (U32)", "RGB (U64)", "Grayscale (U16)"] ("Image Type")
            # "Initialize -- Allocate memory for additional image buffers, if necessary, and perform other one-time initialization steps."
            n20 = call "IMAQ Create"("Border Size"=3, "Image Name"="img0", "Image Type"=w308, "error in (no error)"=w311) -> ("New Image"=w306:T5, "error out"=w310:errorcluster)  [unwired: 1 in]
            n21 = Unbundle By Name(w302) -> ("___Test___"=w300:i32[])
            n22 = Insert Into Array(array=w300, index=0, new element #1=w299, new element #2=w299, new element #3=w299, new element #4=w299, new element #5=w299) -> (w298:i32[])
            n23 = disable-structure shown="Disabled" {
              disable-tunnel: w298 -> [w317 _]
              frame Disabled {
                w316 = 0 ("index")
                n24 = local read item#-1() -> (w318)
                n25 = Unbundle By Name(w318) -> ("Contours"=w315)
                n26 = Index Array(array=w315, index=w316) -> (element=w314)
                n27 = Unbundle By Name(w314) -> ()  [unwired: 1 out]
                n28 = Bundle By Name(cluster=w314, "Coordinates"=w317) -> (w313:cluster{})
                n29 = Insert Into Array(array=w315, index=w316, new element=w313) -> (w312:cluster{}[])
                n30 = Bundle By Name(cluster=w318, "Global Rectangle"=w317, "Contours"=w312) -> (w319:cluster{})
                n31 = local write item#-1(w319) -> ()
              }
              frame Enabled {
              }
            }
            n32 = Bundle By Name(cluster=w302, "image ref"=w306) -> (w304:T7)
            n33 = Bundle By Name(cluster=w304, "___Test___"=w298) -> (w303:T7)
          }
          frame "(qsm) release" {
            # "Release all front-panel action buttons."
          }
          frame "(qsm) clean up" {
            # "Set the \"Stop webcam\" flag"
            # "Clean up -- Set the \"Stop webcam flag\" and perform other necessary clean-up actions."
            n34 = Bundle By Name(cluster=w326, "qsm.Stop webcam"=TRUE) -> (w325:T7)
          }
          frame "(qsm) shutdown" {
            # "deallocate image buffer memory"
            # "stop the loop"
            # "Shutdown -- Release the state queue, free all image buffer memory, and stop the while-loop structure."
            n35 = Release Queue(queue=w334, error in (no error)=w335) -> (error out=w331:errorcluster)  [unwired: 1 in, 2 out]
            n36 = call "Imaq Dispose"("All Images? (No)"=TRUE, "error in (no error)"=w331) -> ("error out"=w330:errorcluster)  [unwired: 4 in]
          }
          frame "(myRIO) initialize" {
            # "Initialize (myRIO) -- Open channels, configure devices, send setup strings to peripherals, etc."
          }
          frame "(myRIO) clean up" {
            w342 = FALSE ("LED3")
            # "clear the onboard LEDs"
            # "Clean up (myRIO) -- Return myRIO devices and external peripherals to inactive states."
            n37 = xnode "LED 3"("LED0"=w342, "LED1"=w342, "LED2"=w342, "LED3"=w342, "error in (no error)"=w341) -> ("error out"=w340:errorcluster)
          }
          frame "(myRIO) update ports" {
            # "show the button state\non the onboard LEDs"
            # "set the flag"
            # "press the onboard button\nto set the \"save image\" flag"
            # "Update ports (myRIO) -- Read and write onboard devices and external peripherals."
            n38 = xnode "Button"("error in (no error)"=w386) -> ("Value"=w383:bool, "error out"=w385:errorcluster)
            n39 = xnode "LED"("LED0"=w383, "LED1"=w383, "LED2"=w383, "LED3"=w383, "error in (no error)"=w385) -> ("error out"=w384:errorcluster)
          }
          frame "(image) get" {
            # "NOTE:\n1. Use NI-MAX to configure your webcam with the\n     *same* resolution (\"mode\") and attributes as those used \n     to develop your Vision Assistant script, especially if the\n     script depends on absolute ROIs, calibration images, template\n     images, background levels, etc.\n \n     Click \"Save\" to create or update the camera configuration files\n     on the target.\n\n2. Open the Vision Acquisition Express VI above and then\n     select \"Reset to Defaults\" to read the camera configuration\n     files created/updated by NI-MAX in the previous step."
            # "webcam image buffer is\ncreated during the first\ncall of the Vision\nAcquisition Express VI"
            # "Get image -- Retrieve a single webcam image frame and optionally flip the image right side up."
            n40 = Unbundle By Name(w466) -> ("qsm.Stop webcam"=w464:bool)
            n41 = call "Vision Acquisition"("Stop (F)"=w464, "error in"=w465) -> ("Image Out"=w463:T5, "error out"=w462:errorcluster)  [unwired: 22 in, 2 out]
            n42 = case shown="False" FALSE {
              tunnel: w463 -> [w472 w476]
              tunnel: [w472 w475] -> w469
              tunnel: w462 -> [w471 w474]
              tunnel: [w471 w473] -> w468
              frame False {
                # "use webcam image as-is"
              }
              frame True {
                w477 = u32 2 items=["Horizontal", "Vertical", "Central", "1st Diagonal", "2nd Diagonal"] ("Type of Symmetry")
                # "flip image when using\ntable-top camera stand"
                n43 = call "IMAQ Symmetry"("error in (no error)"=w474, "Type of Symmetry"=w477, "Image Src"=w476) -> ("error out"=w473:errorcluster, "Image Dst Out"=w475:T5)  [unwired: 2 in]
              }
            }
            n44 = Bundle By Name(cluster=w466, "qsm.Webcam image ref"=w469) -> (w470:T7)
          }
          frame "(image) analyze" {
            # "Color analyze"
            # "analyzed image buffer is\ncreated during the first\ncall of the Vision\nAssistant Express VI *only*\nwhen \"Create Destination\nImage\" option is enabled"
            # "Analyze image -- Analyze the webcam image with a Vision Assistant script."
            n45 = Unbundle By Name "Unbundle By Name"(w492) -> ("___Test___"=w486:i32[], "qsm.Webcam image ref"=w483:T5)
            n46 = call "Vision Assistant2"("Image In"=w483, "error in"=w480, "ROI Descriptor (Image Mask 1)"="ROI Descriptor COLOR", "ROI Descriptor (Color Classification 1)"="ROI Descriptor COLOR") -> ("Image Out"=w481:T5, "error out"=w479:errorcluster, "Classes (Color Classification 1)"=w482:string[])  [unwired: 21 in]
            n47 = Index Array(array=w482, index=0) -> (element=w490:string)
            n48 = local read "Ball index"() -> (w484:i32)
            n49 = Decimal String To Number(string=w490) -> (number=w485:i32)  [unwired: 2 in, 1 out]
            "Color" <- w485
            n50 = Replace Array Subset(array=w486, new element=w485, index=w484) -> (w487:i32[])
            n51 = Bundle By Name "Bundle By Name"(cluster=w492, "qsm.Analyzed image ref"=w481, "Color class"=w485, "___Test___"=w487) -> (w491:T7)
          }
          frame "(image) show" {
            # "Show image -- Select from among the available image buffers to show on the main image display; use a selector tree or case structure."
            n52 = Unbundle By Name "Unbundle By Name"(w495) -> ("show analyzed"=w494:bool)
            n53 = Unbundle By Name "Unbundle By Name"(w497) -> ("qsm.Analyzed image ref"=w500:T5, "qsm.Webcam image ref"=w499:T5)
            n54 = Select(t=w500, s=w494, f=w499) -> (s? t:f=→"image display":T5)
          }
          frame "(ball) Shape detection" {
            # "Shape detection"
            # "Expansion State A"
            n55 = Unbundle By Name(w515) -> ("qsm.Webcam image ref"=w517:T5)
            n56 = call "Vision Assistant"("Image In"=w517, "error in"=w518, "Circle Descriptor (Shape Detection 1)"="Circle Descriptor (Shape Detection 1)") -> ("Image Out"=w516:T5, "error out"=w513:errorcluster, "Circles Calibrated (Shape Detection 1)"=w511:T2, "Number of Matches (Shape Detection 1)"=→"Number of Matches (Shape Detection 1)":i32)  [unwired: 21 in]
            "Circles Calibrated (Shape Detection 1)" <- w511
            n57 = Index Array(array=w511, index=0) -> (element=w507:T23)
            n58 = Unbundle By Name(w507) -> ("Position"=w506:cluster{"X":sgl, "Y":sgl}, "Radius"=→"CircleRadius":dbl)
            n59 = Unbundle(w506) -> ("X"=w505:sgl, "Y"=w504:sgl)
            n60 = To Double Precision Float(number=w505) -> (double precision float=→"curX":dbl)
            n61 = To Double Precision Float(number=w504) -> (double precision float=→"curY":dbl)
            n62 = Bundle By Name(cluster=w515, "qsm.Analyzed image ref"=w516) -> (w514:T7)
          }
          frame "(ball) Calc ball indx" {
            n63 = local read "Circles Calibrated (Shape Detection 1)"() -> (w523:T2)
            n64 = control-ref of="Ball index"() -> (w525:refnum<vi>)
            n65 = control-ref of="Number of Matches (Shape Detection 1)"() -> (w526:refnum<vi>)
            n66 = local read "curX"() -> (w522:dbl)
            n67 = local read "curY"() -> (w521:dbl)
            n68 = To Single Precision Float(number=w522) -> (single precision float=w520:sgl)
            n69 = To Single Precision Float(number=w521) -> (single precision float=w519:sgl)
            n70 = call "Ball Index (SubVI).vi"("cur pos Y"=w519, "cur pos X"=w520, "Circles Calibrated (Shape Detection 1)"=w523, "Ball index"="Ball index", "reference in"=w525, "Digital in"=w526) -> ()  [unwired: 4 in]
          }
          frame "(ball) Calculate ROI" {
            n71 = local read "Number of Matches (Shape Detection 1)"() -> (w540:i32)
            n72 = Greater Than 0?(x=w540) -> (x > 0?=w537:bool)
            n73 = local read "curX"() -> (w539:dbl)
            n74 = local read "curY"() -> (w538:dbl)
            n75 = control-ref of="CircleRadius"() -> (w532:refnum<vi>)
            n76 = local read "ROI Descriptor COLOR"() -> (w530:T1)
            n77 = call "Ball ROI (SubVI).vi"("ROI Descriptor COLOR Mask"=w530, "divider (circle)"="divider (circle)", "curY"=w538, "curX"=w539, "Boolean"=w537, "Digital in"=w532) -> ("x1"=→"x1 (circle)":i32, "y0"=→"y0 (circle)":i32, "x0"=→"x0 (circle)":i32, "ROI Descriptor COLOR Mask out"=w531:T1, "y1"=→"y1 (circle)":i32)  [unwired: 1 in]
            n78 = local write "ROI Descriptor COLOR"(w531) -> ()
            "error out 2" <- w544
          }
          frame "X align" {
            # "Align"
            # "Expansion State B"
            n79 = flat-sequence {
              frame #0 {
                w548 = FALSE ("X is in range")
                n80 = local write "X is in range"(w548) -> ()
                n81 = local write "Y is in range"(w548) -> ()
              }
              frame #1 {
                n82 = control-ref of="Align X - t, Y - f"() -> (w551:refnum<vi>)
                n83 = control-ref of="X is in range"() -> (w550:refnum<vi>)
                n84 = control-ref of="Y is in range"() -> (w549:refnum<vi>)
                n85 = local read "curX"() -> (w561:dbl)
                n86 = local read "curY"() -> (w558:dbl)
                n87 = call "Ball Align(SubVI).vi"("align (t-x/f-y)"=w551, "defY"="defY", "defX"="defX", "Range"="Range", "x is in range"=w550, "y is in range"=w549, "curX"=w561, "curY"=w558, "Align X - t, Y - f"="Align X - t, Y - f") -> ("Boolean"=w552:bool, "Boolean 4"=w555:bool, "Boolean 3"=w554:bool, "Boolean 2"=w553:bool, "x_is_in_range"=→"X is in range":bool, "y_is_in_range"=→"Y is in range":bool)  [unwired: 1 in]
                n88 = local write "Left+"(w552) -> ()
                n89 = local write "Left-"(w555) -> ()
                n90 = local write "Right+"(w554) -> ()
                n91 = local write "Right-"(w553) -> ()
              }
            }
          }
          frame "Wait" {
            w574 = FALSE
            # "Expansion State D"
            n92 = local write "Left-"(w574) -> ()
            n93 = local write "Left+"(w574) -> ()
            n94 = local write "Right+"(w574) -> ()
            n95 = local write "Right-"(w574) -> ()
            n96 = local read "X is in range"() -> (w572:bool)
            n97 = local read "Y is in range"() -> (w571:bool)
            n98 = And(x=w572, y=w571) -> (x .and. y?=w573:bool)
            n99 = case shown="False" w573 {
              tunnel: w570 -> [w579 w584]
              tunnel: [w579 w584] -> w569
              tunnel: w568 -> [w578 w582]
              tunnel: [w576 w581] -> w567
              tunnel: w566 -> [w577 w583]
              tunnel: [w577 w583] -> w565
              tunnel: w564 -> [_ _]
              frame False {
                n100 = Bundle By Name(cluster=w578, "Shape - t, Color - f"=T20."Align") -> (w576:T6)
              }
              frame True {
                n101 = Bundle By Name(cluster=w582, "Shape - t, Color - f"=T20."Clear") -> (w581:T6)
              }
            }
          }
          frame "Grab" {
            # "Expansion State E"
            n102 = call "Grab (SubVI).vi"("error in (no error)"=w588, "M+ (onGrab)"="M+ (onGrab)", "grab time (ms)"="grab time (ms)") -> ("error out"=w587:errorcluster)  [unwired: 8 in]
          }
          frame "(pattern) Find Square" {
            # "analyzed image buffer is\ncreated during the first\ncall of the Vision\nAssistant Express VI *only*\nwhen \"Create Destination\nImage\" option is enabled"
            # "Expansion State F"
            n103 = Unbundle By Name "Unbundle By Name"(w593) -> ("qsm.Webcam image ref"=w598:T5)
            n104 = call "Vision Assistant3"("Image In"=w598, "error in"=w594) -> ("Image Out"=w591:T5, "error out"=w595:errorcluster, "Calibrated Matches (Geometric Matching 1)"=→"Calibrated Matches (Geometric Matching 1)":T3[], "Number of Matches (Geometric Matching 1)"=→"Number of Matches (Geometric Matching 1)":i32)  [unwired: 22 in]
            n105 = Bundle By Name(cluster=w593, "qsm.Analyzed image ref"=w591) -> (w592:T7)
          }
          frame "(pattern) Calculate ROI" {
            # "Expansion State G"
            n106 = local read "Number of Matches (Geometric Matching 1)"() -> (w610:i32)
            n107 = local read "Calibrated Matches (Geometric Matching 1)"() -> (w609:T3[])
            n108 = Unbundle By Name(w612) -> ("ROI Descriptor (Image Mask 1).Contours"=w602:T24)
            n109 = Greater Than 0?(x=w610) -> (x > 0?=w614:bool)
            n110 = call "Pattern ROI (SubVI).vi"("y"="y", "Boolean"=w614, "Calibrated Matches (Geometric Matching 1)"=w609, "Contours in"=w602) -> ("Numeric 4"=→"y1":i32, "Numeric 3"=→"x1":i32, "Numeric"=→"y0":i32, "Scale"=→"Scale":sgl, "Numeric 2"=→"x0":i32, "Contours out"=w601:T24)  [unwired: 2 in]
            n111 = Bundle By Name(cluster=w612, "ROI Descriptor (Image Mask 1).Contours"=w601) -> (w600:T7)
          }
          frame "(pattern) Analyze pattern" {
            n112 = Unbundle By Name(w620) -> ("qsm.Webcam image ref"=w624:T5, "ROI Descriptor (Image Mask 1)"=w618:T1)
            n113 = call "Vision Assistant4"("Image In"=w624, "error in"=w622, "ROI Descriptor (Image Mask 1)"=w618, "ROI Descriptor (Particle Classification 1)"=w618) -> ("Image Out"=w623:T5, "error out"=w621:errorcluster, "Class (Particle Classification 1)"=w616:string)  [unwired: 21 in]
            "Class (Particle Classification 1)" <- w616
            n114 = Decimal String To Number(string=w616) -> (number=w615:i32)  [unwired: 2 in, 1 out]
            n115 = Bundle By Name(cluster=w620, "qsm.Analyzed image ref"=w623, "Pattern class"=w615) -> (w619:T7)
          }
          frame "(joystick) Joystick control" {
            n116 = call "Joystick control (SubVI).vi"() -> ("Boolean 6"=w631:bool, "Boolean 8"=w633:bool, "Boolean 7"=w632:bool, "Boolean 5"=w630:bool, "Boolean 2"=w626:bool, "Boolean"=w625:bool, "Boolean 3"=w627:bool, "Boolean 4"=w628:bool)  [unwired: 4 in]
            n117 = local write "Right+"(w628) -> ()
            n118 = local write "Right-"(w625) -> ()
            n119 = local write "G-"(w630) -> ()
            n120 = local write "M-"(w632) -> ()
            n121 = local write "M+"(w633) -> ()
            n122 = local write "G+"(w631) -> ()
            n123 = local write "Left+"(w626) -> ()
            n124 = local write "Left-"(w627) -> ()
          }
          frame "Wait for button" {
            n125 = while {
              stop <- w642 stop-if-true
              n126 = local read "Stop"() -> (w641:bool)
              n127 = Or(x="Look at ball", y=w641) -> (x .or. y?=w642:bool)
            }
            n128 = local write "Look at ball"(FALSE ("Look at ball")) -> ()
          }
        }
        n129 = Merge Errors(w47, w46) -> (w27:errorcluster)
        n130 = xnode "LED"("LED0"="x = y?", "error in (no error)"=w27) -> ("error out"=w26:errorcluster)
        n131 = Unbundle By Name(w22) -> ("Pattern class"=w25:i32, "___Test___"=w17:i32[])
        "___Test___" <- w17
        n132 = Merge Errors(w18, w26) -> (w51:errorcluster)
        n133 = local read "Number of Matches (Shape Detection 1)"() -> (w24:i32)
        n134 = local read "Ball index"() -> (w15:i32)
        n135 = Index Array(array=w17, index=w15) -> (element=w16:i32)
        n136 = Equal?(x=w25, y=w16) -> (x = y?=w19:bool)
        n137 = local write "x = y?"(w19) -> ()
        n138 = Greater Than 0?(x=w24) -> (x > 0?=w23:bool)
        n139 = case shown="True" w23 {
          tunnel: [w62 w68] -> w21
          tunnel: w22 -> [w61 w68]
          frame False {
            n140 = Unbundle By Name(w61) -> ("___Test___"=w58:i32[])
            n141 = for {
              N: 5 -> [w66]
              tunnel: [w67] -> w60
              tunnel: w58 -> [w64]
              n142 = Decrement(x=w66) -> (x-1=w65:i32)
              n143 = Replace Array Subset(array=w64, new element=20, index=w65) -> (w67:i32[])
            }
            n144 = Bundle By Name(cluster=w61, "___Test___"=w60) -> (w62:T7)
          }
          frame True {
          }
        }
      }
    }
    frame #1 {
      w646 = FALSE ("X is in range")
      n145 = call <vilib>:"Simple Error Handler.vi"("error in (no error)"=w645) -> ("error out"=w644:errorcluster)  [unwired: 4 in, 4 out]
      "error out" <- w644
      n146 = local write "X is in range"(w646) -> ()
      n147 = local write "Y is in range"(w646) -> ()
      n148 = local write "Stop"(w646) -> ()
      n149 = local write "Look at ball"(w646) -> ()
      n150 = local write "x = y?"(w646) -> ()
      n151 = local write "Ball index"(1 ("Ball index")) -> ()
    }
  }
  n152 = call <vilib>:"Reset myRIO.vi"("error in (no error)"=w7) -> ()  [unwired: 10 in, 1 out]
